vi "DblMonoPMDCurrentScanSM correction.vi"() -> ()   [LabVIEW 2009]
uses:
  <vilib>/DAQmx/create/channels.llb/DAQmx Create Channel (AI-Voltage-Basic).vi
  <vilib>/DAQmx/create/channels.llb/DAQmx Create Channel (AO-Voltage-Basic).vi
  <vilib>/DAQmx/write.llb/DAQmx Write (Analog DBL 1Chan 1Samp).vi
  <vilib>/DAQmx/read.llb/DAQmx Read (Analog 1D DBL 1Chan NSamp).vi
  <vilib>/DAQmx/configure/timing.llb/DAQmx Timing (Sample Clock).vi
  <vilib>/DAQmx/read.llb/DAQmx Read (Analog 1D DBL NChan 1Samp).vi
  <vilib>/DAQmx/write.llb/DAQmx Write (Analog 2D DBL NChan NSamp).vi
  <vilib>/Utility/file.llb/Write To Spreadsheet File (DBL).vi
  <vilib>/Analysis/NI_AALBase.lvlib
panel:
  out "element 2":dbl=0.0010963909721584337
  out "element":dbl=0.0027987340470992097
  out "number of samples written per channel":u32=999
  out "Waveform Chart  Y":dbl[](graph)=[0.0007739084085187373, 0.0007735634433916032, 0.0007732184782644691, 0.0007728735131373351, 0.0007725285480102011, 0.0007721835828830671, 0.0007718386177559331, 0.0007714936526287989, 0.0007711486875016649, 0.0007708037223745309, 0.0007704587572473969, 0.0007701137921202628, 0.0007697688269931288, 0.0007694238618659948, 0.0007690788967388608, 0.0007687339316117267, 0.0007683889664845927, 0.0007680440013574586, 0.0007676990362303246, 0.0007673540711031905, 0.0007670091059760565, 0.0007666641408489225, 0.0007663191757217885, 0.0007659742105946543, 0.0007656292454675203, 0.0007652842803403863, 0.0007649393152132523, 0.0007645943500861182, 0.0007642493849589842, 0.0007639044198318502, 0.0007635594547047162, 0.0007632144895775822, 0.000762869524450448, 0.000762524559323314, 0.00076217959419618, 0.000761834629069046, 0.0007614896639419119, 0.0007611446988147779, 0.0007607997336876438, 0.0007604547685605098, 0.0007601098034333757, 0.0007597648383062417, 0.0007594198731791077, 0.0007590749080519737, 0.0007587299429248396, 0.0007583849777977056, 0.0007580400126705716, 0.0007576950475434376, 0.0007573500824163034, 0.0007570051172891694, 0.0007566601521620354, 0.0007563151870349014, 0.0007559702219077673, 0.0007556252567806332, 0.0007552802916534992, 0.0007549353265263652, 0.0007545903613992311, 0.0007542453962720971, 0.0007539004311449631, 0.0007535554660178291, 0.0007532105008906951, 0.000752865535763561, 0.000752520570636427, 0.0007521756055092929, 0.0007518306403821589, 0.0007514856752550248, 0.0007511407101278908, 0.0007507957450007568, 0.0007504507798736228, 0.0007501058147464887, 0.0007497608496193547, 0.0007494158844922206, 0.0007490709193650866, 0.0007487259542379525, 0.0007483809891108185, 0.0007480360239836845, 0.0007476910588565505, 0.0007473460937294165, 0.0007470011286022824, 0.0007466561634751484, 0.0007463111983480143, 0.0007459662332208803, 0.0007456212680937462, 0.0007452763029666122, 0.0007449313378394782, 0.0007445863727123442, 0.00074424140758521, 0.000743896442458076, 0.000743551477330942, 0.000743206512203808, 0.0007428615470766739, 0.0007425165819495399, 0.0007421716168224059, 0.0007418266516952719, 0.0007414816865681378, 0.0007411367214410038, 0.0007407917563138697, 0.0007404467911867357, 0.0007401018260596016, 0.0007397568609324676, 0.0007394118958053336, 0.0007390669306781995, 0.0007387219655510654, 0.0007383770004239314, 0.0007380320352967974, 0.0007376870701696634, 0.0007373421050425294, 0.0007369971399153953, 0.0007366521747882613, 0.0007363072096611273, 0.0007359622445339933, 0.0007356172794068591, 0.0007352723142797251, 0.0007349273491525911, 0.0007345823840254571, 0.000734237418898323, 0.000733892453771189, 0.0007335474886440549, 0.0007332025235169209, 0.0007328575583897868, 0.0007325125932626528, 0.0007321676281355188, 0.0007318226630083848, 0.0007314776978812507, 0.0007311327327541167, 0.0007307877676269827, 0.0007304428024998486, 0.0007300978373727145, 0.0007297528722455805, 0.0007294079071184465, 0.0007290629419913125, 0.0007287179768641785, 0.0007283730117370443, 0.0007280280466099103, 0.0007276830814827763, 0.0007273381163556423, 0.0007269931512285082, 0.0007266481861013742, 0.0007263032209742402, 0.0007259582558471062, 0.0007256132907199721, 0.0007252683255928381, 0.000724923360465704, 0.00072457839533857, 0.0007242334302114359, 0.0007238884650843019, 0.0007235434999571679, 0.0007231985348300339, 0.0007228535697028998, 0.0007225086045757657, 0.0007221636394486317, 0.0007218186743214977, 0.0007214737091943636, 0.0007211287440672296, 0.0007207837789400956, 0.0007204388138129616, 0.0007200938486858276, 0.0007197488835586934, 0.0007194039184315594, 0.0007190589533044254, 0.0007187139881772914, 0.0007183690230501573, 0.0007180240579230233, 0.0007176790927958893, 0.0007173341276687553, 0.0007169891625416211, 0.0007166441974144871, 0.0007162992322873531, 0.0007159542671602191, 0.000715609302033085, 0.000715264336905951, 0.000714919371778817, 0.000714574406651683, 0.0007142294415245488, 0.0007138844763974148, 0.0007135395112702808, 0.0007131945461431468, 0.0007128495810160127, 0.0007125046158888787, 0.0007121596507617447, 0.0007118146856346106, 0.0007114697205074765, 0.0007111247553803425, 0.0007107797902532085, 0.0007104348251260745, 0.0007100898599989405, 0.0007097448948718064, 0.0007093999297446724, 0.0007090549646175384, 0.0007087099994904044, 0.0007083650343632702, 0.0007080200692361362, 0.0007076751041090022, 0.0007073301389818682, 0.0007069851738547341, 0.0007066402087276001, 0.000706295243600466, 0.000705950278473332, 0.0007056053133461979, 0.0007052603482190639, 0.0007049153830919299, 0.0007045704179647959, 0.0007042254528376618, 0.0007038804877105278, 0.0007035355225833938, 0.0007031905574562597, 0.0007028455923291256, 0.0007025006272019916, 0.0007021556620748576, 0.0007018106969477236, 0.0007014657318205896, 0.0007011207666934554, 0.0007007758015663214, 0.0007004308364391874, 0.0007000858713120534, 0.0006997409061849193, 0.0006993959410577853, 0.0006990509759306513, 0.0006987060108035173, 0.0006983610456763832, 0.0006980160805492492, 0.0006976711154221151, 0.0006973261502949811, 0.000696981185167847, 0.000696636220040713, 0.000696291254913579, 0.000695946289786445, 0.0006956013246593108, 0.0006952563595321769, 0.0006949113944050428, 0.0006945664292779088, 0.0006942214641507747, 0.0006938764990236407, 0.0006935315338965067, 0.0006931865687693727, 0.0006928416036422385, 0.0006924966385151046, 0.0006921516733879705, 0.0006918067082608365, 0.0006914617431337025, 0.0006911167780065684, 0.0006907718128794344, 0.0006904268477523004, 0.0006900818826251663, 0.0006897369174980323, 0.0006893919523708982, 0.0006890469872437642, 0.0006887020221166302, 0.0006883570569894961, 0.0006880120918623621, 0.0006876671267352281, 0.000687322161608094, 0.0006869771964809599, 0.0006866322313538259, 0.0006862872662266919, 0.0006859423010995579, 0.0006855973359724238, 0.0006852523708452898, 0.0006849074057181558, 0.0006845624405910217, 0.0006842174754638876, 0.0006838725103367536, 0.0006835275452096196, 0.0006831825800824856, 0.0006828376149553516, 0.0006824926498282175, 0.0006821476847010835, 0.0006818027195739495, 0.0006814577544468154, 0.0006811127893196814, 0.0006807678241925473, 0.0006804228590654133, 0.0006800778939382793, 0.0006797329288111451, 0.0006793879636840112, 0.0006790429985568771, 0.0006786980334297431, 0.000678353068302609, 0.000678008103175475, 0.000677663138048341, 0.000677318172921207, 0.000676973207794073, 0.0006766282426669389, 0.0006762832775398049, 0.0006759383124126708, 0.0006755933472855367, 0.0006752483821584027, 0.0006749034170312687, 0.0006745584519041347, 0.0006742134867770005, 0.0006738685216498666, 0.0006735235565227325, 0.0006731785913955985, 0.0006728336262684645, 0.0006724886611413304, 0.0006721436960141964, 0.0006717987308870624, 0.0006714537657599284, 0.0006711088006327942, 0.0006707638355056603, 0.0006704188703785262, 0.0006700739052513922, 0.0006697289401242581, 0.0006693839749971241, 0.0006690390098699901, 0.0006686940447428561, 0.0006683490796157219, 0.000668004114488588, 0.0006676591493614539, 0.0006673141842343199, 0.0006669692191071858, 0.0006666242539800518, 0.0006662792888529178, 0.0006659343237257838, 0.0006655893585986496, 0.0006652443934715157, 0.0006648994283443816, 0.0006645544632172476, 0.0006642094980901136, 0.0006638645329629795, 0.0006635195678358455, 0.0006631746027087115, 0.0006628296375815774, 0.0006624846724544433, 0.0006621397073273093, 0.0006617947422001753, 0.0006614497770730413, 0.0006611048119459072, 0.0006607598468187732, 0.0006604148816916392, 0.0006600699165645051, 0.000659724951437371, 0.000659379986310237, 0.000659035021183103, 0.000658690056055969, 0.000658345090928835, 0.0006580001258017009, 0.0006576551606745669, 0.0006573101955474328, 0.0006569652304202987, 0.0006566202652931647, 0.0006562753001660307, 0.0006559303350388967, 0.0006555853699117627, 0.0006552404047846286, 0.0006548954396574946, 0.0006545504745303605, 0.0006542055094032265, 0.0006538605442760924, 0.0006535155791489584, 0.0006531706140218244, 0.0006528256488946904, 0.0006524806837675562, 0.0006521357186404223, 0.0006517907535132882, 0.0006514457883861542, 0.0006511008232590201, 0.0006507558581318861, 0.0006504108930047521, 0.0006500659278776181, 0.000649720962750484, 0.00064937599762335, 0.000649031032496216, 0.0006486860673690819, 0.0006483411022419479, 0.0006479961371148138, 0.0006476511719876798, 0.0006473062068605458, 0.0006469612417334117, 0.0006466162766062777, 0.0006462713114791436, 0.0006459263463520096, 0.0006455813812248756, 0.0006452364160977415, 0.0006448914509706075, 0.0006445464858434735, 0.0006442015207163395, 0.0006438565555892053, 0.0006435115904620714, 0.0006431666253349373, 0.0006428216602078033, 0.0006424766950806692, 0.0006421317299535352, 0.0006417867648264012, 0.0006414417996992672, 0.000641096834572133, 0.0006407518694449991, 0.000640406904317865, 0.000640061939190731, 0.000639716974063597, 0.0006393720089364629, 0.0006390270438093289, 0.0006386820786821949, 0.0006383371135550608, 0.0006379921484279268, 0.0006376471833007927, 0.0006373022181736587, 0.0006369572530465247, 0.0006366122879193906, 0.0006362673227922566, 0.0006359223576651226, 0.0006355773925379885, 0.0006352324274108544, 0.0006348874622837204, 0.0006345424971565864, 0.0006341975320294524, 0.0006338525669023183, 0.0006335076017751843, 0.0006331626366480503, 0.0006328176715209162, 0.0006324727063937821, 0.0006321277412666481, 0.0006317827761395141, 0.0006314378110123801, 0.000631092845885246, 0.000630747880758112, 0.000630402915630978, 0.0006300579505038439, 0.0006297129853767099, 0.0006293680202495758, 0.0006290230551224418, 0.0006286780899953078, 0.0006283331248681738, 0.0006279881597410396, 0.0006276431946139057, 0.0006272982294867716, 0.0006269532643596376, 0.0006266082992325035, 0.0006262633341053695, 0.0006259183689782355, 0.0006255734038511015, 0.0006252284387239673, 0.0006248834735968334, 0.0006245385084696993, 0.0006241935433425653, 0.0006238485782154312, 0.0006235036130882972, 0.0006231586479611632, 0.0006228136828340292, 0.000622468717706895, 0.0006221237525797611, 0.000621778787452627, 0.000621433822325493, 0.000621088857198359, 0.0006207438920712249, 0.0006203989269440909, 0.0006200539618169569, 0.0006197089966898228, 0.0006193640315626887, 0.0006190190664355547, 0.0006186741013084207, 0.0006183291361812867, 0.0006179841710541526, 0.0006176392059270186, 0.0006172942407998846, 0.0006169492756727506, 0.0006166043105456164, 0.0006162593454184825, 0.0006159143802913484, 0.0006155694151642144, 0.0006152244500370803, 0.0006148794849099463, 0.0006145345197828123, 0.0006141895546556783, 0.0006138445895285441, 0.0006134996244014102, 0.0006131546592742761, 0.0006128096941471421, 0.000612464729020008, 0.000612119763892874, 0.00061177479876574, 0.000611429833638606, 0.0006110848685114719, 0.0006107399033843378, 0.0006103949382572038, 0.0006100499731300698, 0.0006097050080029358, 0.0006093600428758017, 0.0006090150777486677, 0.0006086701126215337, 0.0006083251474943996, 0.0006079801823672655, 0.0006076352172401315, 0.0006072902521129975, 0.0006069452869858635, 0.0006066003218587294, 0.0006062553567315954, 0.0006059103916044614, 0.0006055654264773273, 0.0006052204613501932, 0.0006048754962230592, 0.0006045305310959252, 0.0006041855659687912, 0.0006038406008416572, 0.000603495635714523, 0.0006031506705873891, 0.000602805705460255, 0.000602460740333121, 0.0006021157752059869, 0.0006017708100788529, 0.0006014258449517189, 0.0006010808798245849, 0.0006007359146974508, 0.0006003909495703168, 0.0006000459844431828, 0.0005997010193160487, 0.0005993560541889146, 0.0005990110890617806, 0.0005986661239346466, 0.0005983211588075126, 0.0005979761936803785, 0.0005976312285532445, 0.0005972862634261105, 0.0005969412982989764, 0.0005965963331718423, 0.0005962513680447083, 0.0005959064029175743, 0.0005955614377904403, 0.0005952164726633063, 0.0005948715075361721, 0.0005945265424090382, 0.0005941815772819041, 0.0005938366121547701, 0.000593491647027636, 0.000593146681900502, 0.000592801716773368, 0.000592456751646234, 0.0005921117865190998, 0.0005917668213919659, 0.0005914218562648318, 0.0005910768911376978, 0.0005907319260105637, 0.0005903869608834297, 0.0005900419957562957, 0.0005896970306291617, 0.0005893520655020275, 0.0005890071003748936, 0.0005886621352477595, 0.0005883171701206255, 0.0005879722049934914, 0.0005876272398663574, 0.0005872822747392234, 0.0005869373096120894, 0.0005865923444849552, 0.0005862473793578212, 0.0005859024142306872, 0.0005855574491035532, 0.0005852124839764192, 0.0005848675188492851, 0.0005845225537221511, 0.0005841775885950171, 0.000583832623467883, 0.0005834876583407489, 0.0005831426932136149, 0.0005827977280864809, 0.0005824527629593469, 0.0005821077978322128, 0.0005817628327050788, 0.0005814178675779448, 0.0005810729024508107, 0.0005807279373236766, 0.0005803829721965426, 0.0005800380070694086, 0.0005796930419422746, 0.0005793480768151405, 0.0005790031116880065, 0.0005786581465608725, 0.0005783131814337384, 0.0005779682163066043, 0.0005776232511794703, 0.0005772782860523363, 0.0005769333209252023, 0.0005765883557980683, 0.0005762433906709341, 0.0005758984255438002, 0.0005755534604166661, 0.0005752084952895321, 0.000574863530162398, 0.000574518565035264, 0.00057417359990813, 0.000573828634780996, 0.0005734836696538618, 0.0005731387045267279, 0.0005727937393995939, 0.0005724487742724598, 0.0005721038091453257, 0.0005717588440181917, 0.0005714138788910577, 0.0005710689137639237, 0.0005707239486367895, 0.0005703789835096556, 0.0005700340183825215, 0.0005696890532553875, 0.0005693440881282534, 0.0005689991230011194, 0.0005686541578739854, 0.0005683091927468514, 0.0005679642276197174, 0.0005676192624925832, 0.0005672742973654493, 0.0005669293322383152, 0.0005665843671111812, 0.0005662394019840471, 0.0005658944368569131, 0.0005655494717297791, 0.0005652045066026451, 0.0005648595414755109, 0.000564514576348377, 0.0005641696112212429, 0.0005638246460941089, 0.0005634796809669748, 0.0005631347158398408, 0.0005627897507127068, 0.0005624447855855728, 0.0005620998204584386, 0.0005617548553313047, 0.0005614098902041706, 0.0005610649250770366, 0.0005607199599499026, 0.0005603749948227685, 0.0005600300296956345, 0.0005596850645685005, 0.0005593400994413664, 0.0005589951343142323, 0.0005586501691870983, 0.0005583052040599643, 0.0005579602389328303, 0.0005576152738056962, 0.0005572703086785622, 0.0005569253435514282, 0.0005565803784242941, 0.00055623541329716, 0.000555890448170026, 0.000555545483042892, 0.000555200517915758, 0.0005548555527886239, 0.0005545105876614899, 0.0005541656225343559, 0.0005538206574072218, 0.0005534756922800877, 0.0005531307271529537, 0.0005527857620258197, 0.0005524407968986857, 0.0005520958317715517, 0.0005517508666444175, 0.0005514059015172836, 0.0005510609363901495, 0.0005507159712630155, 0.0005503710061358814, 0.0005500260410087474, 0.0005496810758816134, 0.0005493361107544794, 0.0005489911456273452, 0.0005486461805002113, 0.0005483012153730772, 0.0005479562502459432, 0.0005476112851188091, 0.0005472663199916751, 0.0005469213548645411, 0.0005465763897374071, 0.0005462314246102729, 0.000545886459483139, 0.0005455414943560049, 0.0005451965292288709, 0.0005448515641017368, 0.0005445065989746028, 0.0005441616338474688, 0.0005438166687203348, 0.0005434717035932006, 0.0005431267384660666, 0.0005427817733389326, 0.0005424368082117986, 0.0005420918430846646, 0.0005417468779575305, 0.0005414019128303965, 0.0005410569477032625, 0.0005407119825761285, 0.0005403670174489943, 0.0005400220523218604, 0.0005396770871947263, 0.0005393321220675923, 0.0005389871569404582, 0.0005386421918133242, 0.0005382972266861902, 0.0005379522615590561, 0.000537607296431922, 0.000537262331304788, 0.000536917366177654, 0.00053657240105052, 0.0005362274359233859, 0.0005358824707962519, 0.0005355375056691179, 0.0005351925405419839, 0.0005348475754148497, 0.0005345026102877157, 0.0005341576451605817, 0.0005338126800334477, 0.0005334677149063137, 0.0005331227497791796, 0.0005327777846520456, 0.0005324328195249116, 0.0005320878543977775, 0.0005317428892706434, 0.0005313979241435094, 0.0005310529590163754, 0.0005307079938892414, 0.0005303630287621073, 0.0005300180636349733, 0.0005296730985078393, 0.0005293281333807052, 0.0005289831682535711, 0.0005286382031264371, 0.0005282932379993031, 0.0005279482728721691, 0.000527603307745035, 0.000527258342617901, 0.000526913377490767, 0.0005265684123636329, 0.0005262234472364988, 0.0005258784821093648, 0.0005255335169822308, 0.0005251885518550968, 0.0005248435867279628, 0.0005244986216008286, 0.0005241536564736947, 0.0005238086913465606, 0.0005234637262194266, 0.0005231187610922925, 0.0005227737959651585, 0.0005224288308380245, 0.0005220838657108905, 0.0005217389005837563, 0.0005213939354566224, 0.0005210489703294883, 0.0005207040052023543, 0.0005203590400752202, 0.0005200140749480862, 0.0005196691098209522, 0.0005193241446938182, 0.000518979179566684, 0.0005186342144395501, 0.0005182892493124161, 0.000517944284185282, 0.000517599319058148, 0.0005172543539310139, 0.0005169093888038799, 0.0005165644236767459, 0.0005162194585496117, 0.0005158744934224777, 0.0005155295282953437, 0.0005151845631682097, 0.0005148395980410757, 0.0005144946329139416, 0.0005141496677868076, 0.0005138047026596736, 0.0005134597375325396, 0.0005131147724054054, 0.0005127698072782715, 0.0005124248421511374, 0.0005120798770240034, 0.0005117349118968693, 0.0005113899467697353, 0.0005110449816426013, 0.0005107000165154672, 0.0005103550513883331, 0.0005100100862611991, 0.0005096651211340651, 0.0005093201560069311, 0.000508975190879797, 0.000508630225752663, 0.000508285260625529, 0.000507940295498395, 0.0005075953303712608, 0.0005072503652441268, 0.0005069054001169928, 0.0005065604349898588, 0.0005062154698627248, 0.0005058705047355906, 0.0005055255396084567, 0.0005051805744813226, 0.0005048356093541886, 0.0005044906442270545, 0.0005041456790999205, 0.0005038007139727865, 0.0005034557488456525, 0.0005031107837185184, 0.0005027658185913844, 0.0005024208534642504, 0.0005020758883371163, 0.0005017309232099822, 0.0005013859580828482, 0.0005010409929557142, 0.0005006960278285802, 0.0005003510627014461, 0.000500006097574312, 0.0004996611324471781, 0.000499316167320044, 0.00049897120219291, 0.0004986262370657759, 0.0004982812719386419, 0.0004979363068115079, 0.0004975913416843739, 0.0004972463765572397, 0.0004969014114301058, 0.0004965564463029717, 0.0004962114811758377, 0.0004958665160487036, 0.0004955215509215696, 0.0004951765857944356, 0.0004948316206673016, 0.0004944866555401674, 0.0004941416904130335, 0.0004937967252858994, 0.0004934517601587654, 0.0004931067950316313, 0.0004927618299044973, 0.0004924168647773633, 0.0004920718996502293, 0.0004917269345230951, 0.0004913819693959611, 0.0004910370042688271, 0.0004906920391416931, 0.000490347074014559, 0.000490002108887425, 0.000489657143760291, 0.000489312178633157, 0.0004889672135060228, 0.0004886222483788888, 0.00048827728325175486, 0.0004879323181246208, 0.00048758735299748676, 0.00048724238787035273, 0.0004868974227432187, 0.0004865524576160847, 0.0004862074924889506, 0.00048586252736181653, 0.00048551756223468256, 0.0004851725971075485, 0.00048482763198041446, 0.00048448266685328044, 0.00048413770172614636, 0.0004837927365990124, 0.0004834477714718783, 0.00048310280634474424, 0.0004827578412176102, 0.0004824128760904762, 0.00048206791096334217, 0.00048172294583620815, 0.00048137798070907407, 0.0004810330155819401, 0.000480688050454806, 0.00048034308532767195, 0.0004799981202005379, 0.0004796531550734039, 0.0004793081899462699, 0.00047896322481913586, 0.0004786182596920018, 0.0004782732945648678, 0.00047792832943773373, 0.00047758336431059966, 0.00047723839918346563, 0.0004768934340563316, 0.0004765484689291976, 0.00047620350380206357, 0.0004758585386749295, 0.0004755135735477954, 0.00047516860842066144, 0.00047482364329352736, 0.00047447867816639334, 0.0004741337130392593, 0.0004737887479121253, 0.0004734437827849913, 0.0004730988176578572, 0.0004727538525307231, 0.00047240888740358915, 0.00047206392227645507, 0.00047171895714932105, 0.000471373992022187, 0.000471029026895053, 0.000470684061767919, 0.0004703390966407849, 0.0004699941315136508, 0.00046964916638651686, 0.0004693042012593828, 0.00046895923613224876, 0.00046861427100511473, 0.0004682693058779807, 0.0004679243407508467, 0.0004675793756237126, 0.00046723441049657853, 0.0004668894453694445, 0.00046654448024231054, 0.00046619951511517647, 0.00046585454998804244, 0.0004655095848609084, 0.0004651646197337744, 0.0004648196546066404, 0.0004644746894795063, 0.0004641297243523722, 0.00046378475922523825, 0.0004634397940981042, 0.00046309482897097015, 0.00046274986384383613, 0.0004624048987167021, 0.0004620599335895681, 0.000461714968462434, 0.00046137000333529993, 0.00046102503820816596, 0.0004606800730810319, 0.00046033510795389786, 0.00045999014282676384, 0.0004596451776996298, 0.0004593002125724958, 0.0004589552474453617, 0.00045861028231822764, 0.0004582653171910936, 0.0004579203520639596, 0.00045757538693682557, 0.00045723042180969154, 0.00045688545668255747, 0.0004565404915554235, 0.0004561955264282894, 0.00045585056130115534, 0.0004555055961740214, 0.0004551606310468873, 0.0004548156659197533, 0.00045447070079261925, 0.0004541257356654852, 0.0004537807705383511, 0.0004534358054112171, 0.00045309084028408316, 0.0004527458751569491, 0.000452400910029815, 0.000452055944902681, 0.00045171097977554696, 0.0004513660146484129, 0.0004510210495212788, 0.0004506760843941448, 0.00045033111926701076, 0.0004499861541398768, 0.0004496411890127427, 0.0004492962238856087, 0.00044895125875847467, 0.0004486062936313406, 0.0004482613285042065, 0.0004479163633770725, 0.00044757139824993847, 0.0004472264331228045, 0.0004468814679956704, 0.0004465365028685364, 0.0004461915377414024, 0.0004458465726142683, 0.0004455016074871342, 0.0004451566423600002, 0.0004448116772328662, 0.0004444667121057322, 0.00044412174697859813, 0.0004437767818514641, 0.0004434318167243301, 0.000443086851597196, 0.00044274188647006193, 0.0004423969213429279, 0.0004420519562157939, 0.0004417069910886598, 0.00044136202596152584, 0.0004410170608343918, 0.0004406720957072578, 0.0004403271305801237, 0.00043998216545298964, 0.0004396372003258556, 0.0004392922351987216, 0.0004389472700715875, 0.00043860230494445355, 0.0004382573398173195, 0.0004379123746901855, 0.0004375674095630514, 0.00043722244443591734, 0.0004368774793087833, 0.0004365325141816493, 0.0004361875490545153, 0.0004358425839273813, 0.00043549761880024723, 0.0004351526536731132, 0.0004348076885459792, 0.0004344627234188451, 0.00043411775829171103, 0.000433772793164577, 0.000433427828037443, 0.0004330828629103089, 0.00043273789778317494, 0.0004323929326560409, 0.0004320479675289069, 0.0004317030024017728, 0.00043135803727463874, 0.0004310130721475047, 0.0004306681070203707, 0.0004303231418932366, 0.00042997817676610265, 0.0004296332116389686, 0.0004292882465118346]
  out "initial y":dbl=0.0007739084085187373
  out "Final Y":dbl=0.0004292882465118346
  out "Waveform Chart X":dbl[](graph)=[0.003443699175398357, 0.0034438293846314775, 0.003443959593864598, 0.0034440898030977185, 0.0034442200123308386, 0.003444350221563959, 0.0034444804307970796, 0.0034446106400301997, 0.00344474084926332, 0.0034448710584964407, 0.0034450012677295612, 0.0034451314769626813, 0.003445261686195802, 0.0034453918954289223, 0.0034455221046620424, 0.003445652313895163, 0.0034457825231282834, 0.0034459127323614035, 0.003446042941594524, 0.0034461731508276445, 0.003446303360060765, 0.003446433569293885, 0.0034465637785270056, 0.003446693987760126, 0.003446824196993246, 0.0034469544062263667, 0.003447084615459487, 0.0034472148246926073, 0.0034473450339257278, 0.0034474752431588483, 0.003447605452391969, 0.003447735661625089, 0.0034478658708582094, 0.00344799608009133, 0.00344812628932445, 0.0034482564985575705, 0.003448386707790691, 0.0034485169170238115, 0.0034486471262569316, 0.003448777335490052, 0.0034489075447231726, 0.0034490377539562926, 0.003449167963189413, 0.0034492981724225337, 0.0034494283816556537, 0.0034495585908887742, 0.0034496888001218948, 0.0034498190093550153, 0.0034499492185881353, 0.003450079427821256, 0.0034502096370543764, 0.0034503398462874964, 0.003450470055520617, 0.0034506002647537374, 0.0034507304739868575, 0.003450860683219978, 0.0034509908924530985, 0.003451121101686219, 0.003451251310919339, 0.0034513815201524596, 0.00345151172938558, 0.0034516419386187, 0.0034517721478518207, 0.0034519023570849412, 0.0034520325663180613, 0.003452162775551182, 0.0034522929847843023, 0.003452423194017423, 0.003452553403250543, 0.0034526836124836634, 0.003452813821716784, 0.003452944030949904, 0.0034530742401830245, 0.003453204449416145, 0.0034533346586492655, 0.0034534648678823856, 0.003453595077115506, 0.0034537252863486266, 0.0034538554955817467, 0.003453985704814867, 0.0034541159140479877, 0.0034542461232811078, 0.0034543763325142283, 0.003454506541747349, 0.0034546367509804693, 0.0034547669602135894, 0.00345489716944671, 0.0034550273786798304, 0.0034551575879129505, 0.003455287797146071, 0.0034554180063791915, 0.0034555482156123116, 0.003455678424845432, 0.0034558086340785526, 0.003455938843311673, 0.003456069052544793, 0.0034561992617779137, 0.003456329471011034, 0.0034564596802441542, 0.0034565898894772747, 0.0034567200987103953, 0.0034568503079435158, 0.003456980517176636, 0.0034571107264097563, 0.003457240935642877, 0.003457371144875997, 0.0034575013541091174, 0.003457631563342238, 0.003457761772575358, 0.0034578919818084785, 0.003458022191041599, 0.0034581524002747195, 0.0034582826095078396, 0.00345841281874096, 0.0034585430279740806, 0.0034586732372072007, 0.0034588034464403212, 0.0034589336556734417, 0.003459063864906562, 0.0034591940741396823, 0.003459324283372803, 0.0034594544926059233, 0.0034595847018390434, 0.003459714911072164, 0.0034598451203052844, 0.0034599753295384045, 0.003460105538771525, 0.0034602357480046455, 0.0034603659572377656, 0.003460496166470886, 0.0034606263757040066, 0.003460756584937127, 0.003460886794170247, 0.0034610170034033677, 0.003461147212636488, 0.0034612774218696083, 0.0034614076311027288, 0.0034615378403358493, 0.00346166804956897, 0.00346179825880209, 0.0034619284680352104, 0.003462058677268331, 0.003462188886501451, 0.0034623190957345715, 0.003462449304967692, 0.003462579514200812, 0.0034627097234339326, 0.003462839932667053, 0.0034629701419001736, 0.0034631003511332937, 0.003463230560366414, 0.0034633607695995347, 0.0034634909788326547, 0.0034636211880657753, 0.0034637513972988958, 0.003463881606532016, 0.0034640118157651363, 0.003464142024998257, 0.0034642722342313774, 0.0034644024434644974, 0.003464532652697618, 0.0034646628619307385, 0.0034647930711638585, 0.003464923280396979, 0.0034650534896300995, 0.00346518369886322, 0.00346531390809634, 0.0034654441173294606, 0.003465574326562581, 0.003465704535795701, 0.0034658347450288217, 0.0034659649542619422, 0.0034660951634950623, 0.003466225372728183, 0.0034663555819613033, 0.003466485791194424, 0.003466616000427544, 0.0034667462096606644, 0.003466876418893785, 0.003467006628126905, 0.0034671368373600255, 0.003467267046593146, 0.003467397255826266, 0.0034675274650593866, 0.003467657674292507, 0.0034677878835256276, 0.0034679180927587477, 0.003468048301991868, 0.0034681785112249887, 0.0034683087204581088, 0.0034684389296912293, 0.00346856913892435, 0.00346869934815747, 0.0034688295573905904, 0.003468959766623711, 0.0034690899758568314, 0.0034692201850899515, 0.003469350394323072, 0.0034694806035561925, 0.0034696108127893126, 0.003469741022022433, 0.0034698712312555536, 0.003470001440488674, 0.003470131649721794, 0.0034702618589549147, 0.003470392068188035, 0.0034705222774211552, 0.0034706524866542758, 0.0034707826958873963, 0.0034709129051205163, 0.003471043114353637, 0.0034711733235867574, 0.003471303532819878, 0.003471433742052998, 0.0034715639512861184, 0.003471694160519239, 0.003471824369752359, 0.0034719545789854795, 0.0034720847882186, 0.00347221499745172, 0.0034723452066848406, 0.003472475415917961, 0.0034726056251510816, 0.0034727358343842017, 0.0034728660436173222, 0.0034729962528504427, 0.003473126462083563, 0.0034732566713166833, 0.003473386880549804, 0.003473517089782924, 0.0034736472990160444, 0.003473777508249165, 0.0034739077174822854, 0.0034740379267154055, 0.003474168135948526, 0.0034742983451816465, 0.0034744285544147666, 0.003474558763647887, 0.0034746889728810076, 0.003474819182114128, 0.003474949391347248, 0.0034750796005803687, 0.003475209809813489, 0.0034753400190466093, 0.00347547022827973, 0.0034756004375128503, 0.0034757306467459704, 0.003475860855979091, 0.0034759910652122114, 0.003476121274445332, 0.003476251483678452, 0.0034763816929115725, 0.003476511902144693, 0.003476642111377813, 0.0034767723206109336, 0.003476902529844054, 0.003477032739077174, 0.0034771629483102947, 0.003477293157543415, 0.0034774233667765357, 0.0034775535760096558, 0.0034776837852427763, 0.0034778139944758968, 0.003477944203709017, 0.0034780744129421374, 0.003478204622175258, 0.0034783348314083784, 0.0034784650406414984, 0.003478595249874619, 0.0034787254591077395, 0.0034788556683408595, 0.00347898587757398, 0.0034791160868071005, 0.0034792462960402206, 0.003479376505273341, 0.0034795067145064616, 0.003479636923739582, 0.0034797671329727022, 0.0034798973422058227, 0.0034800275514389432, 0.0034801577606720633, 0.003480287969905184, 0.0034804181791383043, 0.0034805483883714244, 0.003480678597604545, 0.0034808088068376654, 0.003480939016070786, 0.003481069225303906, 0.0034811994345370265, 0.003481329643770147, 0.003481459853003267, 0.0034815900622363876, 0.003481720271469508, 0.0034818504807026286, 0.0034819806899357487, 0.003482110899168869, 0.0034822411084019897, 0.00348237131763511, 0.0034825015268682303, 0.003482631736101351, 0.003482761945334471, 0.0034828921545675914, 0.003483022363800712, 0.0034831525730338324, 0.0034832827822669525, 0.003483412991500073, 0.0034835432007331935, 0.0034836734099663136, 0.003483803619199434, 0.0034839338284325546, 0.0034840640376656747, 0.003484194246898795, 0.0034843244561319157, 0.003484454665365036, 0.0034845848745981563, 0.0034847150838312768, 0.0034848452930643973, 0.0034849755022975173, 0.003485105711530638, 0.0034852359207637584, 0.0034853661299968784, 0.003485496339229999, 0.0034856265484631195, 0.00348575675769624, 0.00348588696692936, 0.0034860171761624805, 0.003486147385395601, 0.003486277594628721, 0.0034864078038618416, 0.003486538013094962, 0.0034866682223280827, 0.0034867984315612027, 0.0034869286407943232, 0.0034870588500274437, 0.003487189059260564, 0.0034873192684936843, 0.003487449477726805, 0.003487579686959925, 0.0034877098961930454, 0.003487840105426166, 0.0034879703146592864, 0.0034881005238924065, 0.003488230733125527, 0.0034883609423586475, 0.0034884911515917676, 0.003488621360824888, 0.0034887515700580086, 0.0034888817792911287, 0.003489011988524249, 0.0034891421977573697, 0.00348927240699049, 0.0034894026162236103, 0.003489532825456731, 0.0034896630346898513, 0.0034897932439229714, 0.003489923453156092, 0.0034900536623892124, 0.0034901838716223325, 0.003490314080855453, 0.0034904442900885735, 0.003490574499321694, 0.003490704708554814, 0.0034908349177879346, 0.003490965127021055, 0.003491095336254175, 0.0034912255454872957, 0.003491355754720416, 0.0034914859639535367, 0.0034916161731866568, 0.0034917463824197773, 0.0034918765916528978, 0.003492006800886018, 0.0034921370101191384, 0.003492267219352259, 0.003492397428585379, 0.0034925276378184994, 0.00349265784705162, 0.0034927880562847405, 0.0034929182655178605, 0.003493048474750981, 0.0034931786839841016, 0.0034933088932172216, 0.003493439102450342, 0.0034935693116834626, 0.0034936995209165827, 0.0034938297301497032, 0.0034939599393828237, 0.0034940901486159442, 0.0034942203578490643, 0.003494350567082185, 0.0034944807763153053, 0.0034946109855484254, 0.003494741194781546, 0.0034948714040146664, 0.0034950016132477865, 0.003495131822480907, 0.0034952620317140275, 0.003495392240947148, 0.003495522450180268, 0.0034956526594133886, 0.003495782868646509, 0.003495913077879629, 0.0034960432871127497, 0.00349617349634587, 0.0034963037055789907, 0.003496433914812111, 0.0034965641240452313, 0.003496694333278352, 0.003496824542511472, 0.0034969547517445924, 0.003497084960977713, 0.003497215170210833, 0.0034973453794439535, 0.003497475588677074, 0.0034976057979101945, 0.0034977360071433146, 0.003497866216376435, 0.0034979964256095556, 0.0034981266348426757, 0.003498256844075796, 0.0034983870533089167, 0.0034985172625420368, 0.0034986474717751573, 0.0034987776810082778, 0.0034989078902413983, 0.0034990380994745184, 0.003499168308707639, 0.0034992985179407594, 0.0034994287271738794, 0.003499558936407, 0.0034996891456401205, 0.003499819354873241, 0.003499949564106361, 0.0035000797733394816, 0.003500209982572602, 0.003500340191805722, 0.0035004704010388426, 0.003500600610271963, 0.0035007308195050832, 0.0035008610287382037, 0.0035009912379713242, 0.0035011214472044448, 0.003501251656437565, 0.0035013818656706853, 0.003501512074903806, 0.003501642284136926, 0.0035017724933700464, 0.003501902702603167, 0.003502032911836287, 0.0035021631210694075, 0.003502293330302528, 0.0035024235395356485, 0.0035025537487687686, 0.003502683958001889, 0.0035028141672350096, 0.0035029443764681297, 0.00350307458570125, 0.0035032047949343707, 0.003503335004167491, 0.0035034652134006113, 0.003503595422633732, 0.0035037256318668523, 0.0035038558410999724, 0.003503986050333093, 0.0035041162595662134, 0.0035042464687993335, 0.003504376678032454, 0.0035045068872655745, 0.003504637096498695, 0.003504767305731815, 0.0035048975149649356, 0.003505027724198056, 0.003505157933431176, 0.0035052881426642967, 0.003505418351897417, 0.0035055485611305373, 0.0035056787703636578, 0.0035058089795967783, 0.0035059391888298988, 0.003506069398063019, 0.0035061996072961394, 0.00350632981652926, 0.00350646002576238, 0.0035065902349955005, 0.003506720444228621, 0.003506850653461741, 0.0035069808626948615, 0.003507111071927982, 0.0035072412811611026, 0.0035073714903942226, 0.003507501699627343, 0.0035076319088604637, 0.0035077621180935837, 0.0035078923273267042, 0.0035080225365598247, 0.003508152745792945, 0.0035082829550260653, 0.003508413164259186, 0.0035085433734923063, 0.0035086735827254264, 0.003508803791958547, 0.0035089340011916674, 0.0035090642104247875, 0.003509194419657908, 0.0035093246288910285, 0.003509454838124149, 0.003509585047357269, 0.0035097152565903896, 0.00350984546582351, 0.00350997567505663, 0.0035101058842897507, 0.003510236093522871, 0.0035103663027559913, 0.003510496511989112, 0.0035106267212222323, 0.003510756930455353, 0.003510887139688473, 0.0035110173489215934, 0.003511147558154714, 0.003511277767387834, 0.0035114079766209545, 0.003511538185854075, 0.003511668395087195, 0.0035117986043203156, 0.003511928813553436, 0.0035120590227865566, 0.0035121892320196767, 0.003512319441252797, 0.0035124496504859177, 0.0035125798597190378, 0.0035127100689521583, 0.0035128402781852788, 0.003512970487418399, 0.0035131006966515194, 0.00351323090588464, 0.0035133611151177604, 0.0035134913243508805, 0.003513621533584001, 0.0035137517428171215, 0.0035138819520502415, 0.003514012161283362, 0.0035141423705164826, 0.003514272579749603, 0.003514402788982723, 0.0035145329982158437, 0.003514663207448964, 0.0035147934166820842, 0.0035149236259152047, 0.0035150538351483252, 0.0035151840443814453, 0.003515314253614566, 0.0035154444628476863, 0.003515574672080807, 0.003515704881313927, 0.0035158350905470474, 0.003515965299780168, 0.003516095509013288, 0.0035162257182464085, 0.003516355927479529, 0.003516486136712649, 0.0035166163459457696, 0.00351674655517889, 0.0035168767644120106, 0.0035170069736451307, 0.003517137182878251, 0.0035172673921113717, 0.003517397601344492, 0.0035175278105776123, 0.003517658019810733, 0.0035177882290438533, 0.0035179184382769734, 0.003518048647510094, 0.0035181788567432144, 0.0035183090659763345, 0.003518439275209455, 0.0035185694844425755, 0.0035186996936756956, 0.003518829902908816, 0.0035189601121419366, 0.003519090321375057, 0.003519220530608177, 0.0035193507398412977, 0.003519480949074418, 0.0035196111583075383, 0.0035197413675406588, 0.0035198715767737793, 0.0035200017860068994, 0.00352013199524002, 0.0035202622044731404, 0.003520392413706261, 0.003520522622939381, 0.0035206528321725015, 0.003520783041405622, 0.003520913250638742, 0.0035210434598718626, 0.003521173669104983, 0.003521303878338103, 0.0035214340875712236, 0.003521564296804344, 0.0035216945060374647, 0.0035218247152705847, 0.0035219549245037052, 0.0035220851337368258, 0.003522215342969946, 0.0035223455522030663, 0.003522475761436187, 0.0035226059706693074, 0.0035227361799024274, 0.003522866389135548, 0.0035229965983686684, 0.0035231268076017885, 0.003523257016834909, 0.0035233872260680295, 0.0035235174353011496, 0.00352364764453427, 0.0035237778537673906, 0.003523908063000511, 0.003524038272233631, 0.0035241684814667517, 0.0035242986906998722, 0.0035244288999329923, 0.003524559109166113, 0.0035246893183992333, 0.0035248195276323534, 0.003524949736865474, 0.0035250799460985944, 0.003525210155331715, 0.003525340364564835, 0.0035254705737979555, 0.003525600783031076, 0.003525730992264196, 0.0035258612014973166, 0.003525991410730437, 0.003526121619963557, 0.0035262518291966777, 0.003526382038429798, 0.0035265122476629187, 0.0035266424568960388, 0.0035267726661291593, 0.00352690287536228, 0.0035270330845954, 0.0035271632938285204, 0.003527293503061641, 0.0035274237122947614, 0.0035275539215278815, 0.003527684130761002, 0.0035278143399941225, 0.0035279445492272426, 0.003528074758460363, 0.0035282049676934836, 0.0035283351769266036, 0.003528465386159724, 0.0035285955953928447, 0.003528725804625965, 0.0035288560138590852, 0.0035289862230922057, 0.0035291164323253263, 0.0035292466415584463, 0.003529376850791567, 0.0035295070600246873, 0.0035296372692578074, 0.003529767478490928, 0.0035298976877240484, 0.003530027896957169, 0.003530158106190289, 0.0035302883154234095, 0.00353041852465653, 0.00353054873388965, 0.0035306789431227706, 0.003530809152355891, 0.0035309393615890116, 0.0035310695708221317, 0.0035311997800552522, 0.0035313299892883727, 0.003531460198521493, 0.0035315904077546133, 0.003531720616987734, 0.003531850826220854, 0.0035319810354539744, 0.003532111244687095, 0.0035322414539202154, 0.0035323716631533355, 0.003532501872386456, 0.0035326320816195765, 0.0035327622908526966, 0.003532892500085817, 0.0035330227093189376, 0.0035331529185520577, 0.003533283127785178, 0.0035334133370182987, 0.003533543546251419, 0.0035336737554845393, 0.0035338039647176598, 0.0035339341739507803, 0.0035340643831839004, 0.003534194592417021, 0.0035343248016501414, 0.003534455010883262, 0.003534585220116382, 0.0035347154293495025, 0.003534845638582623, 0.003534975847815743, 0.0035351060570488636, 0.003535236266281984, 0.003535366475515104, 0.0035354966847482247, 0.003535626893981345, 0.0035357571032144657, 0.0035358873124475857, 0.0035360175216807063, 0.0035361477309138268, 0.003536277940146947, 0.0035364081493800673, 0.003536538358613188, 0.003536668567846308, 0.0035367987770794284, 0.003536928986312549, 0.0035370591955456695, 0.0035371894047787895, 0.00353731961401191, 0.0035374498232450305, 0.0035375800324781506, 0.003537710241711271, 0.0035378404509443916, 0.0035379706601775117, 0.003538100869410632, 0.0035382310786437527, 0.0035383612878768732, 0.0035384914971099933, 0.003538621706343114, 0.0035387519155762343, 0.0035388821248093544, 0.003539012334042475, 0.0035391425432755954, 0.003539272752508716, 0.003539402961741836, 0.0035395331709749565, 0.003539663380208077, 0.003539793589441197, 0.0035399237986743176, 0.003540054007907438, 0.003540184217140558, 0.0035403144263736787, 0.003540444635606799, 0.0035405748448399197, 0.0035407050540730398, 0.0035408352633061603, 0.003540965472539281, 0.003541095681772401, 0.0035412258910055214, 0.003541356100238642, 0.003541486309471762, 0.0035416165187048825, 0.003541746727938003, 0.0035418769371711235, 0.0035420071464042436, 0.003542137355637364, 0.0035422675648704846, 0.0035423977741036046, 0.003542527983336725, 0.0035426581925698457, 0.0035427884018029657, 0.0035429186110360862, 0.0035430488202692068, 0.0035431790295023273, 0.0035433092387354473, 0.003543439447968568, 0.0035435696572016884, 0.0035436998664348084, 0.003543830075667929, 0.0035439602849010494, 0.00354409049413417, 0.00354422070336729, 0.0035443509126004105, 0.003544481121833531, 0.003544611331066651, 0.0035447415402997716, 0.003544871749532892, 0.003545001958766012, 0.0035451321679991327, 0.0035452623772322532, 0.0035453925864653737, 0.003545522795698494, 0.0035456530049316143, 0.003545783214164735, 0.003545913423397855, 0.0035460436326309754, 0.003546173841864096, 0.003546304051097216, 0.0035464342603303365, 0.003546564469563457, 0.0035466946787965775, 0.0035468248880296976, 0.003546955097262818, 0.0035470853064959386, 0.0035472155157290587, 0.003547345724962179, 0.0035474759341952997, 0.00354760614342842, 0.0035477363526615403, 0.003547866561894661, 0.0035479967711277813, 0.0035481269803609014, 0.003548257189594022, 0.0035483873988271424, 0.0035485176080602625, 0.003548647817293383, 0.0035487780265265035, 0.003548908235759624, 0.003549038444992744, 0.0035491686542258646, 0.003549298863458985, 0.003549429072692105, 0.0035495592819252257, 0.003549689491158346, 0.0035498197003914662, 0.0035499499096245868, 0.0035500801188577073, 0.0035502103280908278, 0.003550340537323948, 0.0035504707465570684, 0.003550600955790189, 0.003550731165023309, 0.0035508613742564294, 0.00355099158348955, 0.00355112179272267, 0.0035512520019557905, 0.003551382211188911, 0.0035515124204220315, 0.0035516426296551516, 0.003551772838888272, 0.0035519030481213926, 0.0035520332573545127, 0.0035521634665876332, 0.0035522936758207537, 0.0035524238850538742, 0.0035525540942869943, 0.003552684303520115, 0.0035528145127532353, 0.0035529447219863554, 0.003553074931219476, 0.0035532051404525964, 0.0035533353496857165, 0.003553465558918837, 0.0035535957681519575, 0.003553725977385078, 0.003553856186618198, 0.0035539863958513186, 0.003554116605084439, 0.003554246814317559, 0.0035543770235506797, 0.0035545072327838, 0.0035546374420169203, 0.003554767651250041, 0.0035548978604831613, 0.003555028069716282, 0.003555158278949402, 0.0035552884881825224, 0.003555418697415643, 0.003555548906648763, 0.0035556791158818835, 0.003555809325115004, 0.003555939534348124, 0.0035560697435812446, 0.003556199952814365, 0.0035563301620474856, 0.0035564603712806057, 0.003556590580513726, 0.0035567207897468467, 0.0035568509989799667, 0.0035569812082130873, 0.0035571114174462078, 0.0035572416266793283, 0.0035573718359124483, 0.003557502045145569, 0.0035576322543786894, 0.0035577624636118094, 0.00355789267284493, 0.0035580228820780505, 0.0035581530913111705, 0.003558283300544291, 0.0035584135097774115, 0.003558543719010532, 0.003558673928243652, 0.0035588041374767726, 0.003558934346709893, 0.0035590645559430132, 0.0035591947651761337, 0.0035593249744092542, 0.0035594551836423743, 0.003559585392875495, 0.0035597156021086153, 0.003559845811341736, 0.003559976020574856, 0.0035601062298079764, 0.003560236439041097, 0.003560366648274217, 0.0035604968575073375, 0.003560627066740458, 0.003560757275973578, 0.0035608874852066986, 0.003561017694439819, 0.0035611479036729396, 0.0035612781129060597, 0.00356140832213918, 0.0035615385313723007, 0.0035616687406054208, 0.0035617989498385413, 0.003561929159071662, 0.0035620593683047823, 0.0035621895775379024, 0.003562319786771023, 0.0035624499960041434, 0.0035625802052372635, 0.003562710414470384, 0.0035628406237035045, 0.0035629708329366246, 0.003563101042169745, 0.0035632312514028656, 0.003563361460635986, 0.003563491669869106, 0.0035636218791022267, 0.003563752088335347, 0.0035638822975684673, 0.0035640125068015878, 0.0035641427160347083, 0.0035642729252678288, 0.003564403134500949, 0.0035645333437340694, 0.00356466355296719, 0.00356479376220031, 0.0035649239714334304, 0.003565054180666551, 0.003565184389899671, 0.0035653145991327915, 0.003565444808365912, 0.0035655750175990326, 0.0035657052268321526, 0.003565835436065273, 0.0035659656452983936, 0.0035660958545315137, 0.0035662260637646342, 0.0035663562729977547, 0.003566486482230875, 0.0035666166914639953, 0.003566746900697116, 0.0035668771099302363, 0.0035670073191633564, 0.003567137528396477, 0.0035672677376295974, 0.0035673979468627175, 0.003567528156095838, 0.0035676583653289585, 0.003567788574562079, 0.003567918783795199, 0.0035680489930283196, 0.00356817920226144, 0.00356830941149456, 0.0035684396207276807, 0.003568569829960801, 0.0035687000391939213, 0.003568830248427042, 0.0035689604576601623, 0.003569090666893283, 0.003569220876126403, 0.0035693510853595234, 0.003569481294592644, 0.003569611503825764, 0.0035697417130588845, 0.003569871922292005, 0.003570002131525125, 0.0035701323407582456, 0.003570262549991366, 0.0035703927592244866, 0.0035705229684576067, 0.003570653177690727, 0.0035707833869238477, 0.0035709135961569678, 0.0035710438053900883, 0.0035711740146232088, 0.003571304223856329, 0.0035714344330894494, 0.00357156464232257, 0.0035716948515556904, 0.0035718250607888104, 0.003571955270021931, 0.0035720854792550515, 0.0035722156884881715, 0.003572345897721292, 0.0035724761069544126, 0.0035726063161875326, 0.003572736525420653, 0.0035728667346537736, 0.003572996943886894, 0.0035731271531200142, 0.0035732573623531347, 0.0035733875715862552, 0.0035735177808193753, 0.003573647990052496, 0.0035737781992856163]
  out "initial x":dbl=0.003443699175398357
  out "Final x":dbl=0.0035737781992856163
  in  "Volts/pixel":dbl=-0.0002
  out "Xin":dbl=0.0034436991753983574
  out "Yin":dbl=0.0007739084085187373
  in  "Correction":dbl[][](array[numeric])=[[460.0, 480.0, 1.0, -5.0], [480.0, 490.0, 4.0, -6.0], [490.0, 510.0, 4.0, -6.0], [510.0, 530.0, 7.0, -4.0], [530.0, 550.0, 6.0, -4.0], [550.0, 570.0, 11.0, -2.0], [570.0, 590.0, 18.0, 1.0], [590.0, 610.0, 16.0, 1.0], [610.0, 630.0, 22.0, 4.0], [630.0, 650.0, 25.0, 4.0], [650.0, 670.0, 31.0, 4.0], [670.0, 690.0, 24.0, 6.0], [690.0, 710.0, 25.0, 5.0], [710.0, 730.0, 23.0, 3.0], [730.0, 750.0, 19.0, 1.0], [750.0, 780.0, 9.0, 1.0], [780.0, 800.0, 12.0, 0.0]]
  in  "Scan mirrors out":tag="Dev1/ao1:0"
  in  "Scan Mirrors in":tag="Dev1/ai1:2"
  in  "Voltage B":dbl min=-10.0 max=10.0 step=0.1 format="%0.2f"
  in  "Voltage A":dbl min=-10.0 max=10.0 step=0.1 format="%0.2f"
  in  "Output B":tag="Dev1/ao3"
  in  "Output A":tag="Dev1/ao2"
  in  "Input Channel":tag="Dev1/ai6"
  in  "Current":bool
  in  "Power":bool=TRUE
  out "ScanGraph":cluster{dbl[], dbl[]}(graph)={[459.986, 464.987, 469.988, 474.99, 479.99, 484.99, 489.99, 494.99, 499.989, 504.988, 509.986, 514.984, 519.999, 524.996, 529.993, 534.99, 539.986, 544.998, 549.994, 554.99, 559.984, 564.995, 569.99, 574.983, 579.993, 584.986, 589.994, 594.986, 599.995, 604.986, 609.993, 614.983, 619.99, 624.995, 629.985, 634.99, 639.994, 644.999, 649.986, 654.989, 659.992, 664.994, 669.996, 674.997, 679.998, 684.998, 689.983, 694.998, 699.997, 704.996, 709.994, 714.991, 719.988, 724.985, 729.997, 734.993, 739.988, 744.999], [2.1099248219999993e-07, 4.841876133e-06, -1.5273329160000004e-06, 1.7982357982999998e-06, 1.6874433263e-06, 1.7260287571e-06, 4.2421699291e-06, 1.0175213299e-05, 6.336555329000002e-07, 2.8867754744e-06, 9.7345900059e-06, 2.0786917676e-06, 1.262283729e-06, 7.0713391289999995e-06, 2.155351334e-06, -1.245506316000002e-07, 2.1544726345e-06, 2.2136387822e-06, -3.900836119999998e-07, -1.0242116113e-06, 4.19034681275e-06, 1.1503179743e-06, 6.3705236194e-06, 2.431987241e-06, 3.2818190054e-06, 2.2443169879999996e-06, -1.7280163039999998e-07, 3.4131044219999993e-07, -3.1544439536e-06, 4.743758288999999e-07, 2.61580934e-06, 5.132718029e-06, 2.411577974e-06, 2.1582370003e-06, 1.4940037116e-06, -8.682694599999961e-09, 1.1422522415e-06, 1.0737787442000001e-06, -2.239742121e-07, 1.0586110429e-06, 1.0709150784e-06, 1.2884574339000001e-06, 1.0348154043e-06, 4.847385682e-07, 5.49520904e-07, 1.7452527669999997e-07, 4.2117633290000003e-07, 1.07371440189e-06, 2.3799586880999999e-07, 5.871614649e-07, 9.4995538737e-07, -2.8246480500000006e-08, 7.429808617e-08, 6.2026416241e-07, 3.0612814373e-07, 7.033739084e-07, 9.849100580000001e-08, 5.508379621499999e-07]}
  in  "Sensitivity":dbl=1e-09 caption="(A/V)" format="%#_6p"
  out "Readout":dbl=4.29846551e-07 format="%^#_9e"
  in  "Scan Save Path":path
  in  "On":bool=TRUE
  out "Waveform Chart":dbl(graph)=4.29846551e-07
  in  "Save":bool
  in  "Exit":bool
  in  "STOP":bool
  in  "Step Time (sec)":dbl=1.0 min=0.001 max=300.0 step=0.001 format="%.3f"
  in  "Step Size (nm)":dbl=5.0 min=0.1 max=100.0 step=0.1 format="%.1f"
  in  "End":dbl=800.0 min=0.0 max=2000.0 step=0.1 format="%.1f"
  in  "Start":dbl=460.0 min=0.0 max=2000.0 step=0.1 format="%.1f"
  in  "Scan":bool
  in  "Up":bool=TRUE caption="Down"
  in  "Increment (nm)":dbl=10.0 min=0.1 max=2000.0 step=0.1 format="%.1f"
  in  "PMD Settings":T1={"Beam Diameter (mm)"=4.0, "BWIn"=0, "Averaging Rate"=300, "Auto Range"=TRUE} {"Averaging Rate" min=33 max=5000 step=1; "BWIn" items=["HIGH", "LOW"]; "Beam Diameter (mm)" min=1.0 max=9.0 step=0.5}
  in  "Step":bool
  out "Busy":bool
  in  "Send Command":bool
  in  "Command":u16(ring)=1 items=["nm", "goto", "nm/min", "VIS grating", "IR grating"]
  in  "Wavelength (nm)":dbl=745.0 min=0.0 max=2000.0 step=0.1 format="%.1f"
  in  "Scan Speed (nm/min)":dbl=100.0 min=1.0 max=500.0 step=0.1 format="%.1f"
  out "Done?":string="  ok\r\n"
  in  "Send Question":bool
  in  "Ask?":u16(ring) items=["?nm", "?nm/min", "?grating", "?turret", "?gratings"]
  in  "Zero?":bool
  out "PM Error log":string
  out "AUTO?":bool
  out "Zero Value":dbl format="%#.3p"
  out "Rng":string
  in  "Range":i16=1 min=1 max=6 step=1
  in  "Mono Port":refnum<visa-resource-name>="COM11"
  out "IDN String":string="Thorlabs,PM100USB,P2000362,1.3.0\n"
  out "Sensor SN":string="10061433"
  out "Sensor Name":string="S120C"
  out "Reply":string=" 744.999 nm  ok\r\n" caption="Mono Response"
  # "Range Settings"
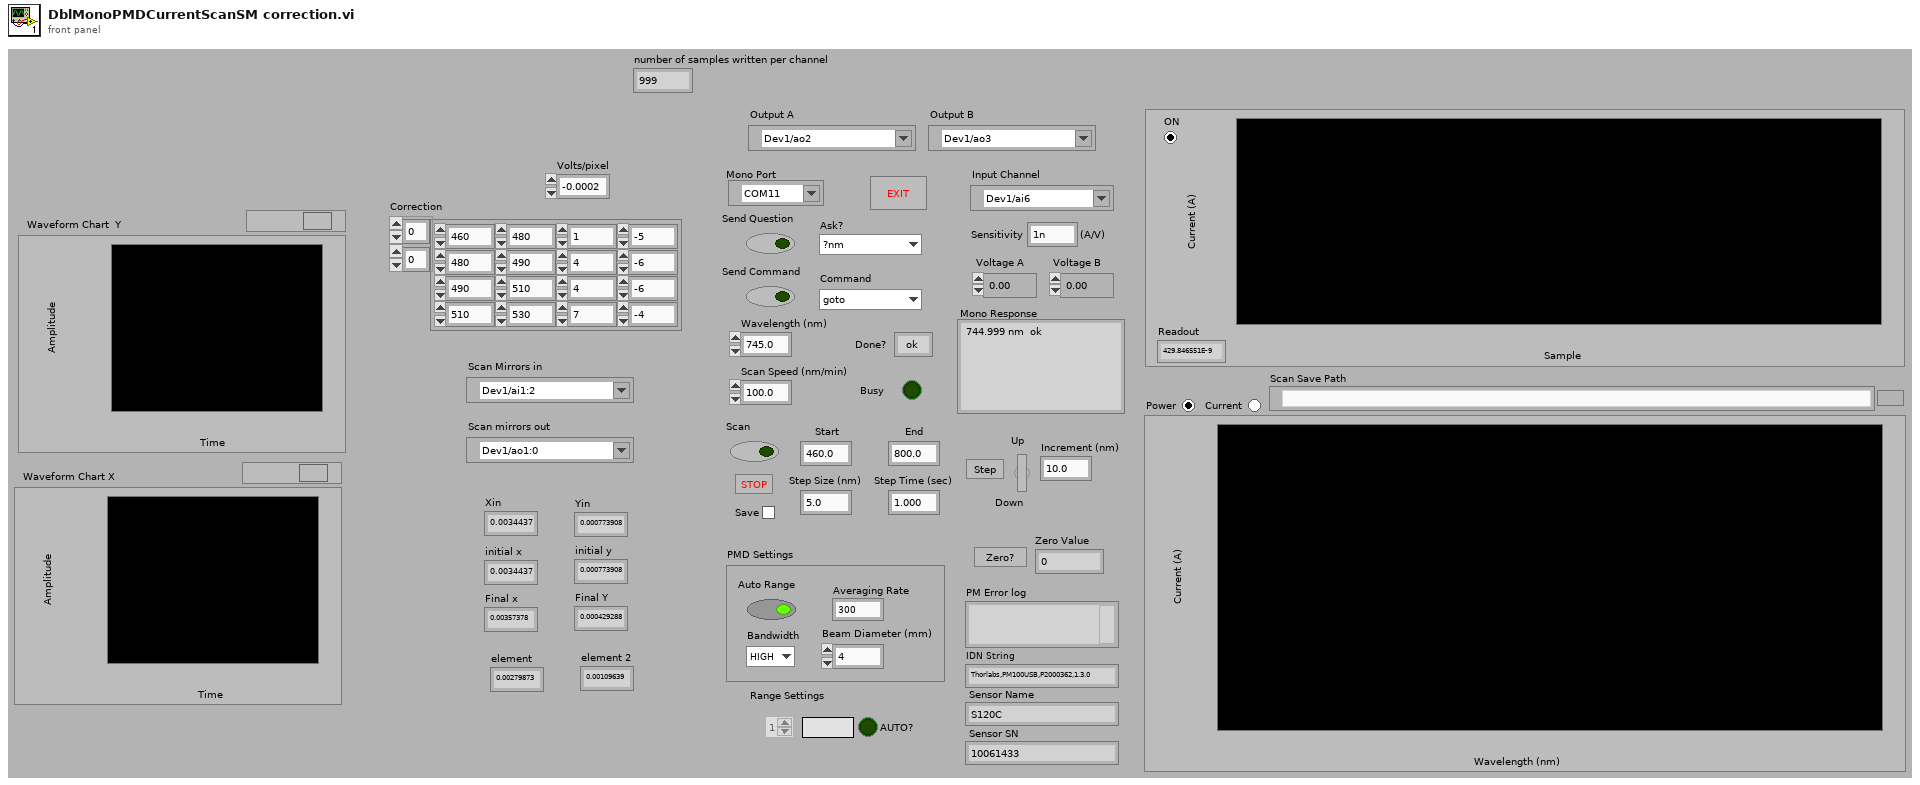
[diagram p1: front panel]
types:
  T1 = cluster{"Beam Diameter (mm)":dbl, "BWIn":u16, "Averaging Rate":i32, "Auto Range":bool}
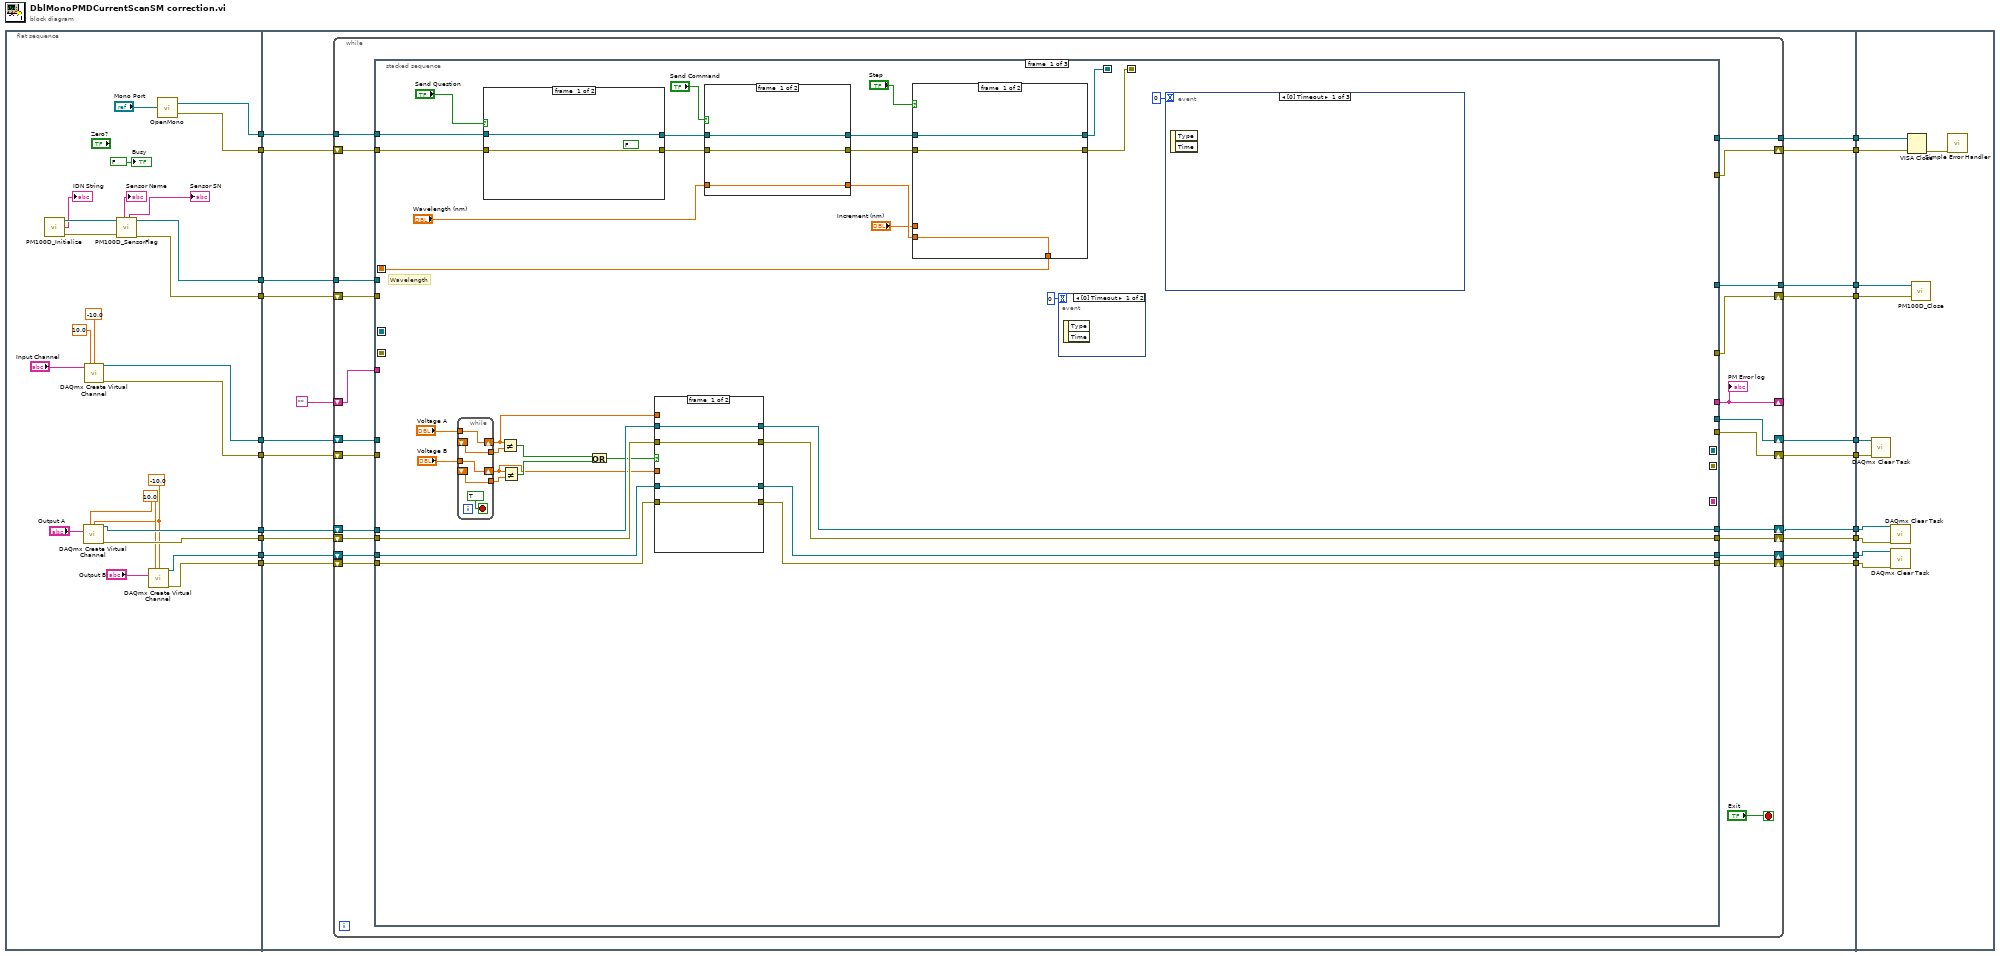
[diagram p0: block diagram]
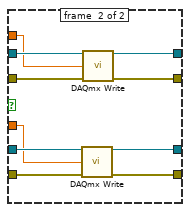
[diagram p2: hidden frame]
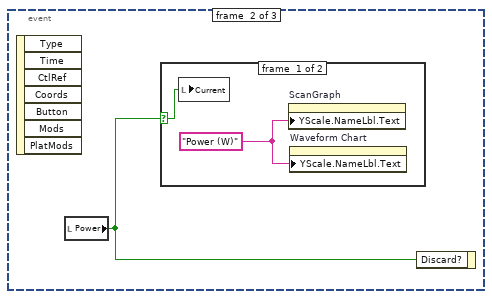
[diagram p3: hidden frame]
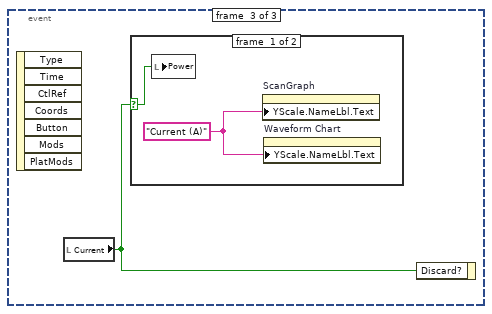
[diagram p5: hidden frame]
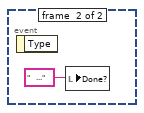
[diagram p7: hidden frame]
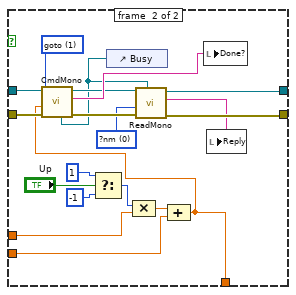
[diagram p8: hidden frame]
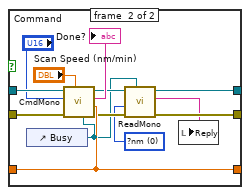
[diagram p9: hidden frame]
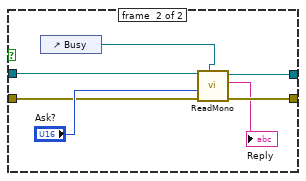
[diagram p10: hidden frame]
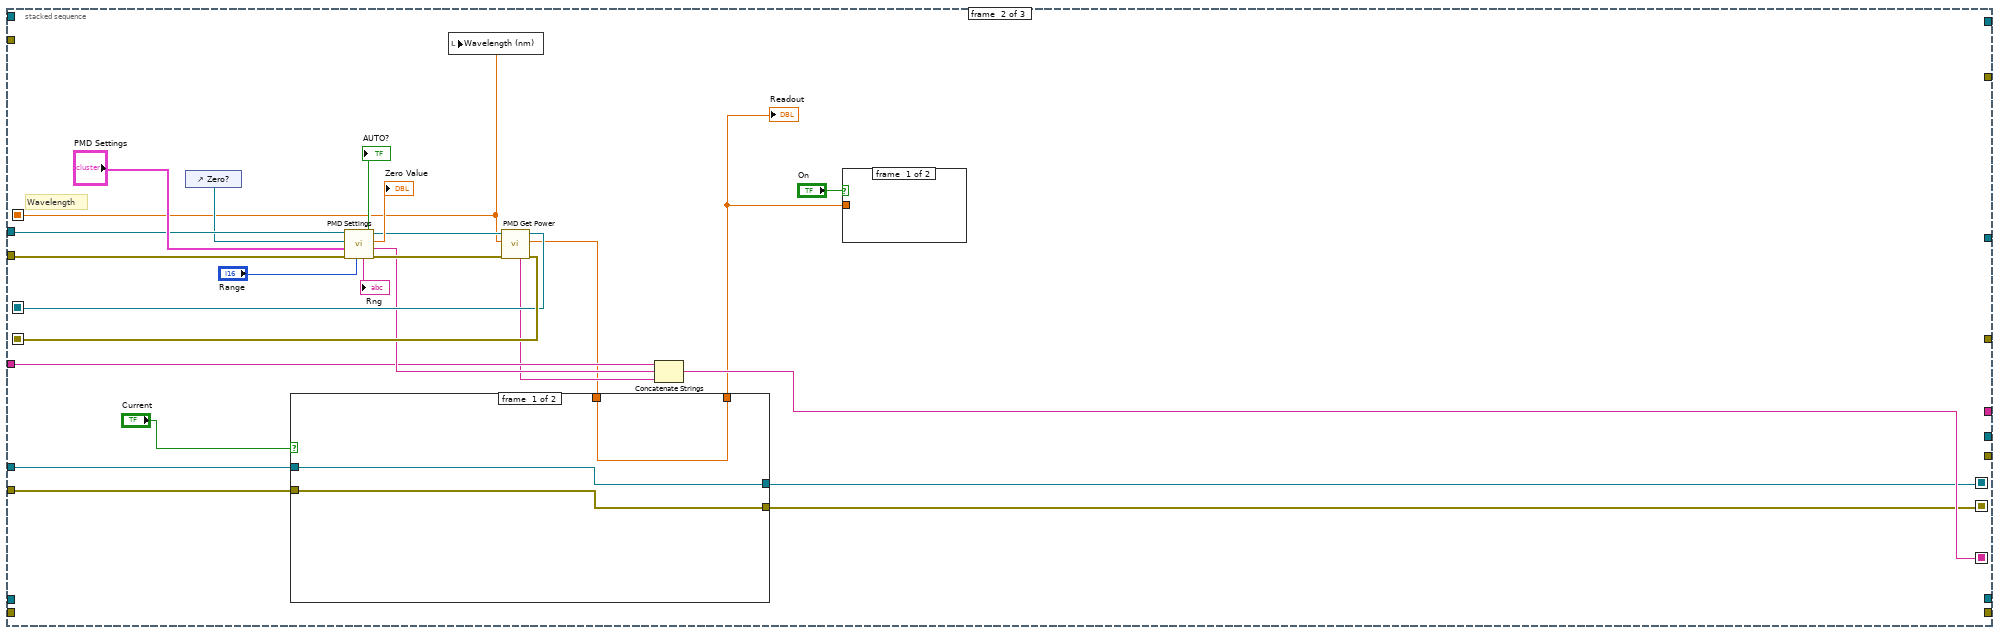
[diagram p11: hidden frame]
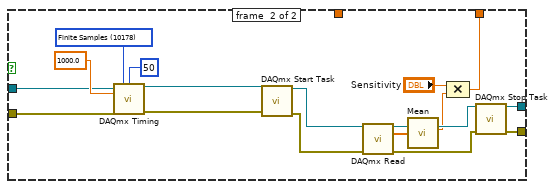
[diagram p12: hidden frame]
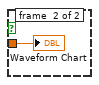
[diagram p13: hidden frame]
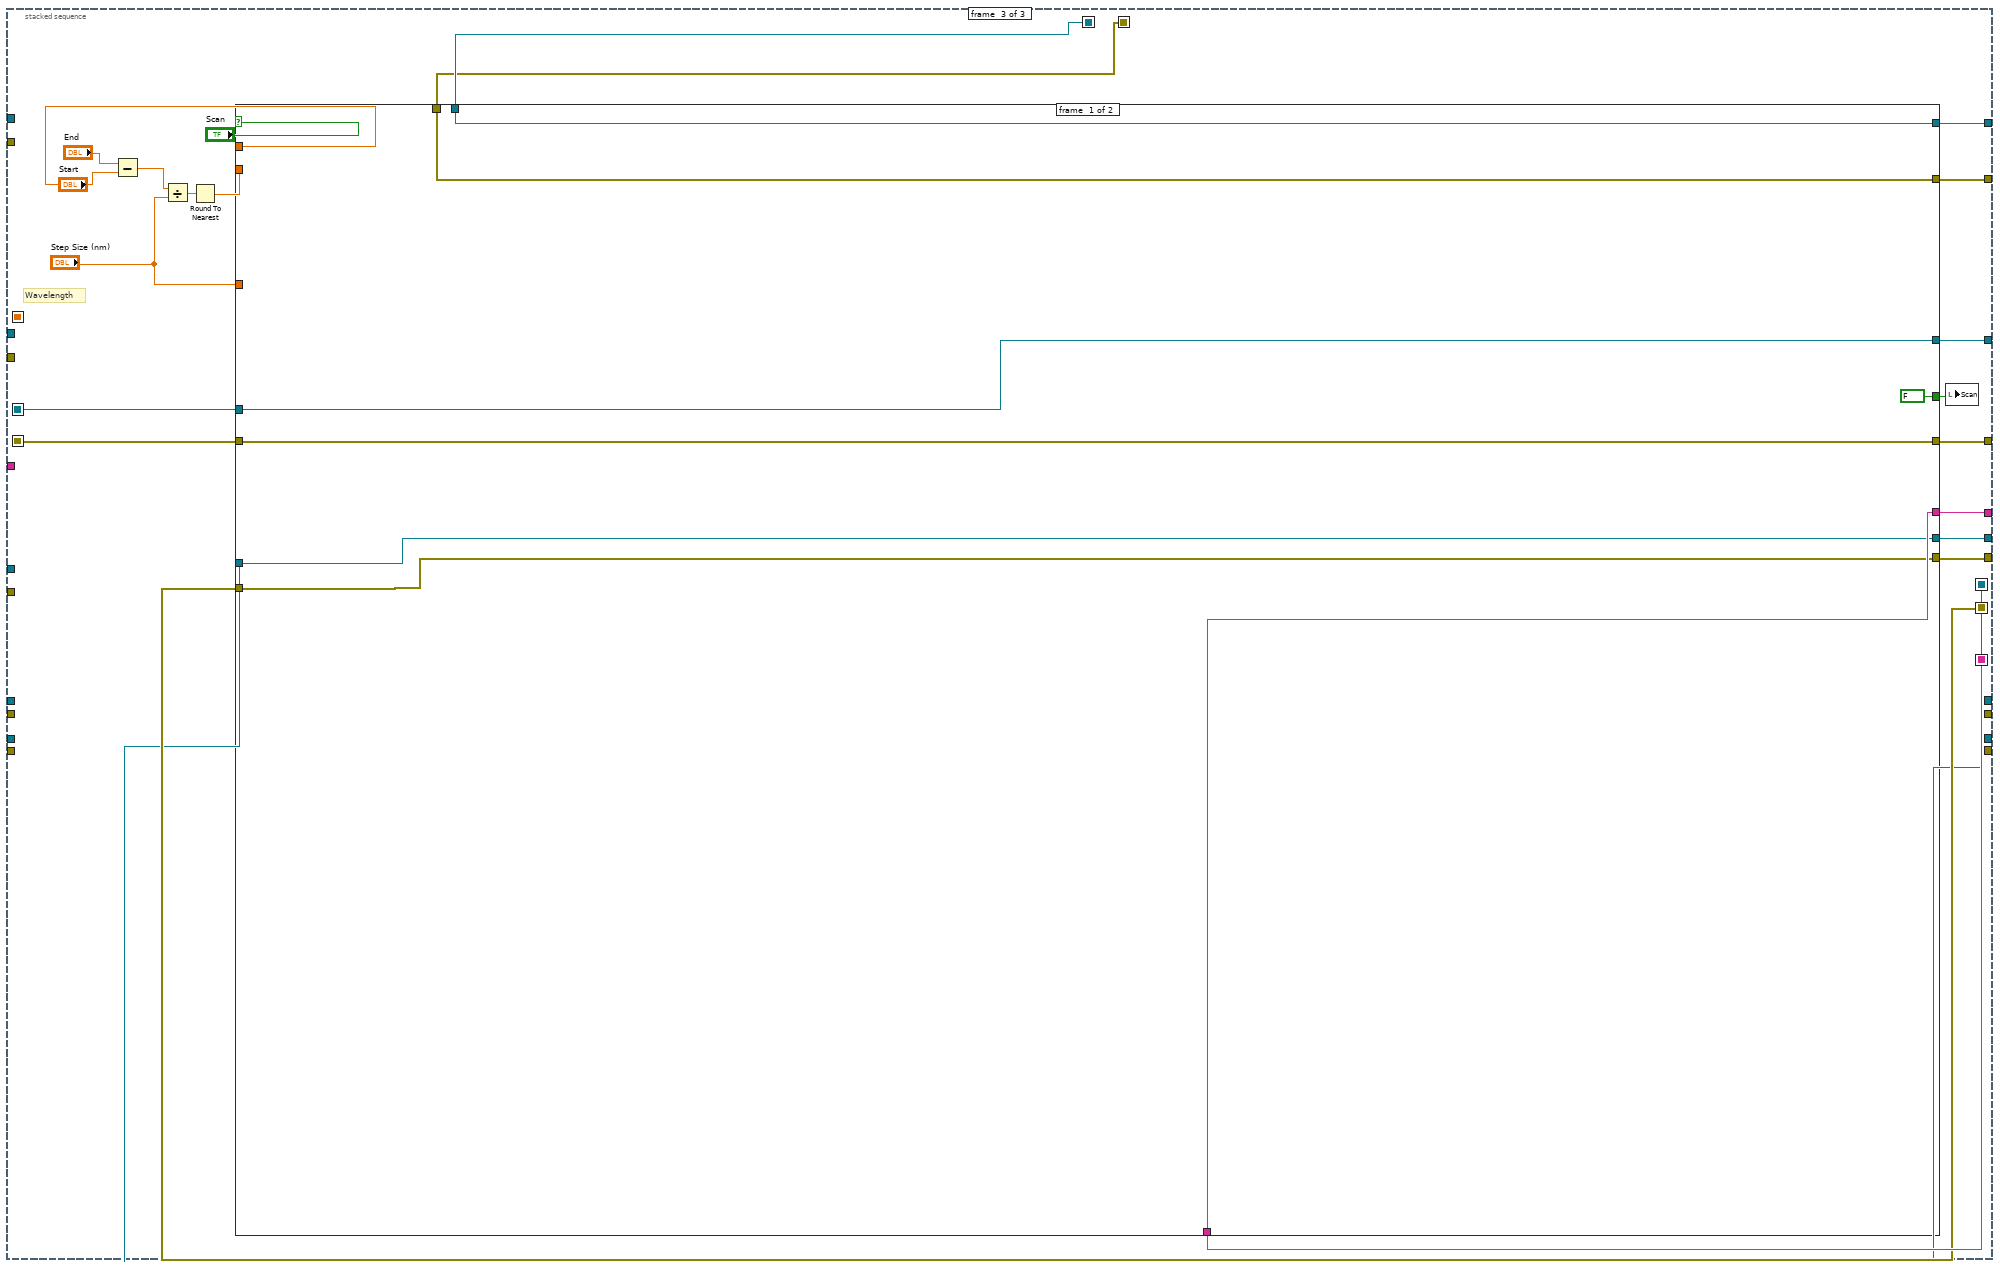
[diagram p14: hidden frame]
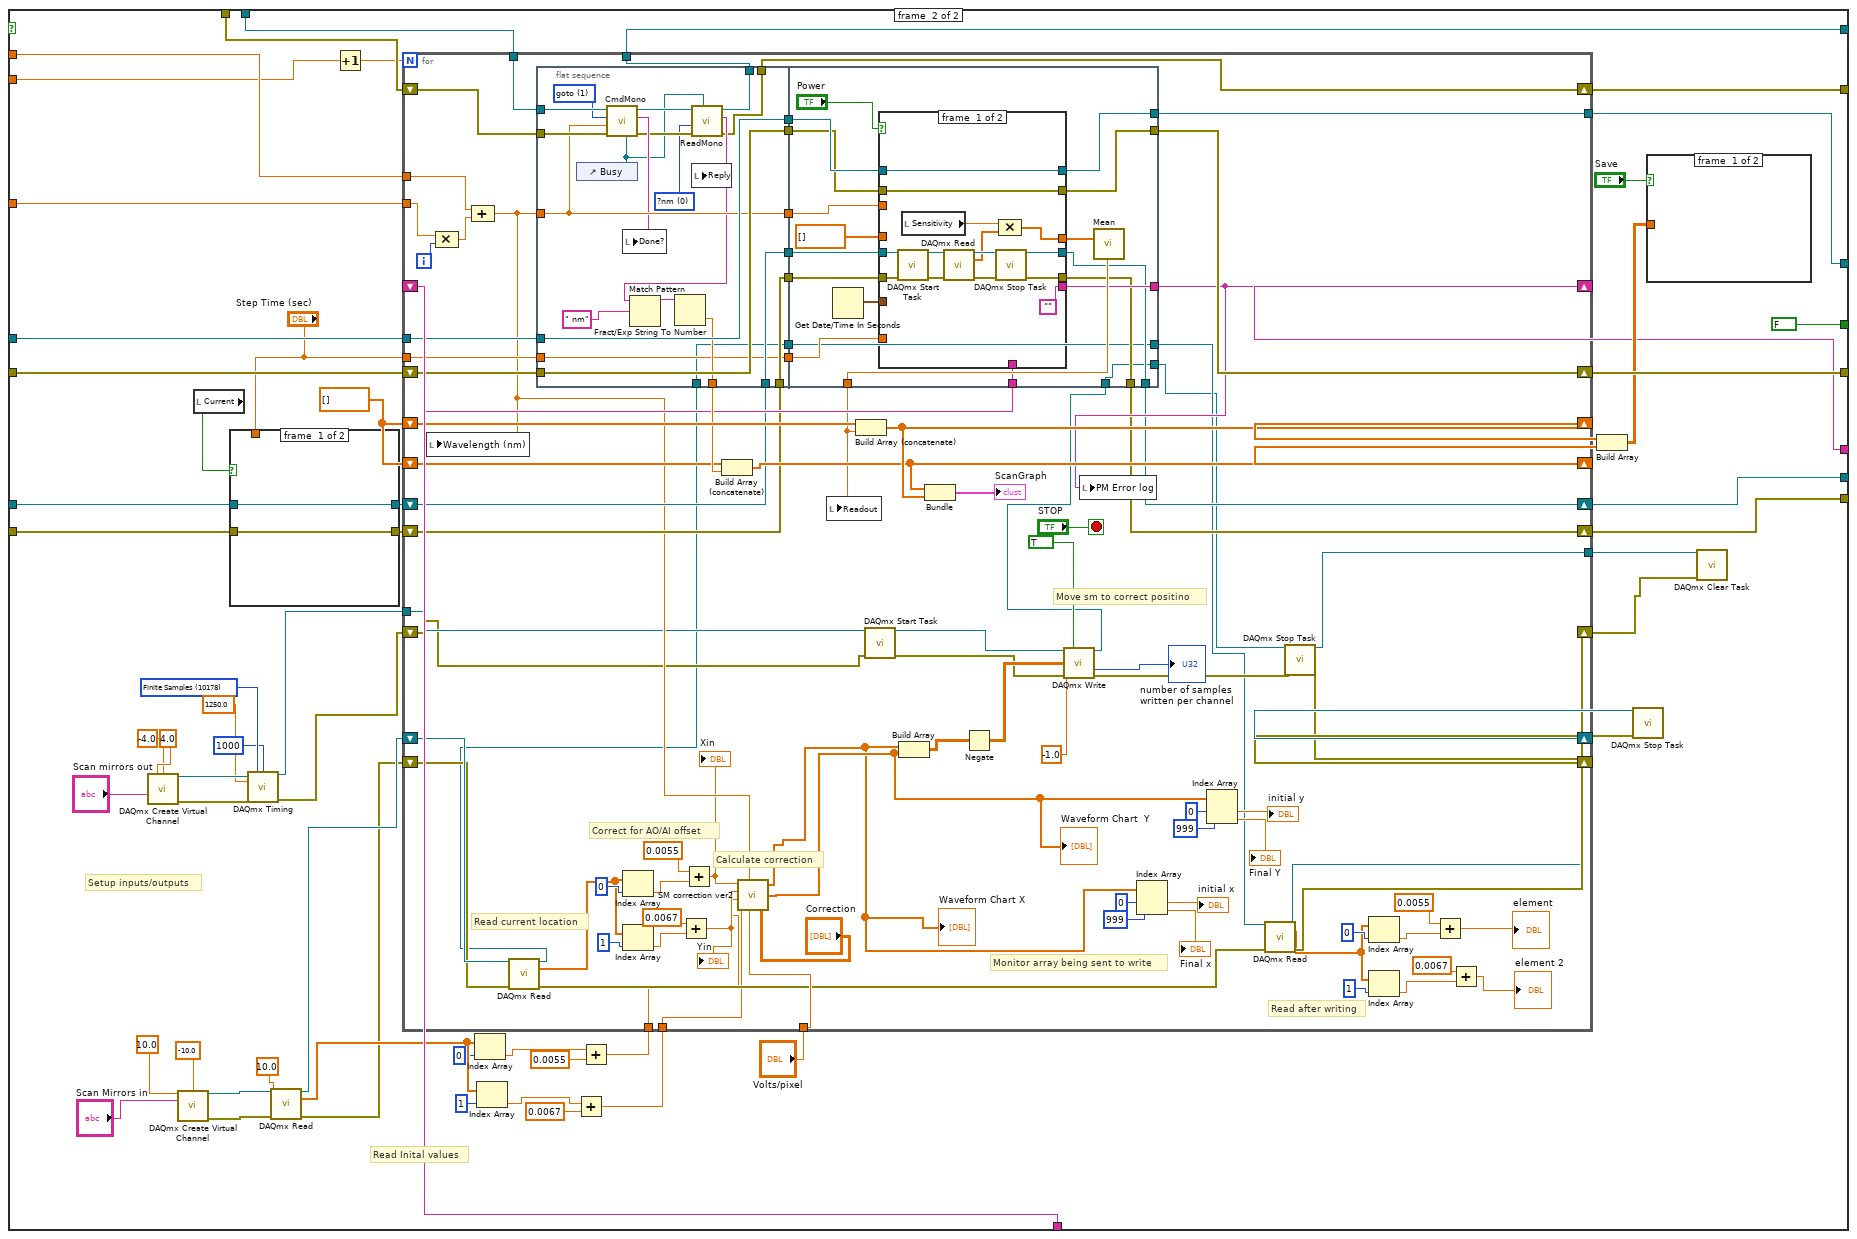
[diagram p15: hidden frame]
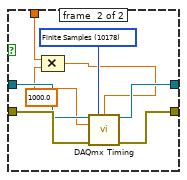
[diagram p16: hidden frame]
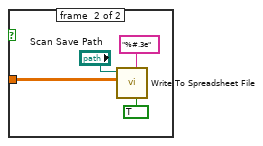
[diagram p17: hidden frame]
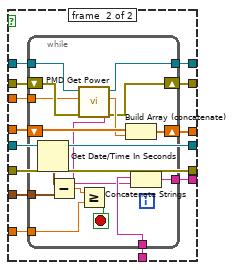
[diagram p18: hidden frame]
diagram:
  n1 = flat-sequence {
    tunnel: [w39] -> w20
    tunnel: [w38] -> w19
    tunnel: [w37] -> w18
    tunnel: [w36] -> w17
    tunnel: [w23] -> w12
    tunnel: [w24] -> w9
    tunnel: [w29] -> w8
    tunnel: [w30] -> w7
    tunnel: [w28] -> w6
    tunnel: [w27] -> w5
    tunnel: w20 -> [w64]
    tunnel: w19 -> [w65]
    tunnel: w18 -> [w63]
    tunnel: w17 -> [w62]
    tunnel: [w61] -> w16
    tunnel: [w60] -> w15
    tunnel: [w59] -> w14
    tunnel: [w58] -> w13
    tunnel: w12 -> [w55]
    tunnel: [w46] -> w11
    tunnel: [w45] -> w10
    tunnel: w9 -> [w56]
    tunnel: w8 -> [w54]
    tunnel: w7 -> [w53]
    tunnel: w6 -> [w52]
    tunnel: w5 -> [w51]
    tunnel: [w47] -> w4
    tunnel: [w48] -> w3
    tunnel: [w49] -> w2
    tunnel: [w50] -> w1
    tunnel: w16 -> [w526]
    tunnel: w15 -> [w525]
    tunnel: w14 -> [w524]
    tunnel: w13 -> [w523]
    tunnel: w11 -> [w521]
    tunnel: w10 -> [w522]
    tunnel: w4 -> [w520]
    tunnel: w3 -> [w519]
    tunnel: w2 -> [w518]
    tunnel: w1 -> [w517]
    frame #0 {
      w25 = -10.0 ("minimum value")
      w26 = 10.0 ("maximum value")
      n2 = call "PM100D_Initialize.vi"() -> ("error out"=w43:errorcluster, "Instrument"=→"IDN String":string, "VISA out"=w44:refnum<visa-resource-name>)  [unwired: 2 in, 1 out]
      n3 = call-poly <vilib>:"DAQmx Create Virtual Channel.vi"("maximum value"=w26, "minimum value"=w25, "physical channels"="Output A") -> ("task out"=w30:refnum<k21>, "error out"=w29:errorcluster)  [unwired: 11 in]
      n4 = call-poly <vilib>:"DAQmx Create Virtual Channel.vi"("maximum value"=10.0, "minimum value"=-10.0, "physical channels"="Input Channel") -> ("task out"=w24:refnum<k21>, "error out"=w23:errorcluster)  [unwired: 11 in]
      n5 = call "PM100D_SensorFlag.vi"("error in (no error)"=w43, "VISA in"=w44) -> ("error out"=w39:errorcluster, "VISA out"=w38:refnum<visa-resource-name>, "sn"=→"Sensor SN":string, "name"=→"Sensor Name":string)  [unwired: 2 in, 4 out]
      n6 = call-poly <vilib>:"DAQmx Create Virtual Channel.vi"("maximum value"=w26, "minimum value"=w25, "physical channels"="Output B") -> ("task out"=w27:refnum<k21>, "error out"=w28:errorcluster)  [unwired: 11 in]
      n7 = call "OpenMono.vi"("Mono Port"="Mono Port") -> ("VISA resource name out"=w37:refnum<visa-resource-name>, "error out"=w36:errorcluster)
      "Busy" <- FALSE ("Busy")
    }
    frame #1 {
      n8 = while {
        tunnel: w65 -> [w86]
        tunnel: w63 -> [w88]
        tunnel: [w83] -> w60
        tunnel: [w81] -> w58
        shift-right: [w80] -> w59
        shift-left: w64 -> [w85]
        shift-right: [w82] -> w61
        shift-left: w62 -> [w87]
        shift-right: [w78] -> _
        shift-left: "" -> [w79]
        shift-right: [w67] -> w45
        shift-left: w55 -> [w76]
        shift-right: [w66] -> w46
        shift-left: w56 -> [w77]
        shift-right: [w68] -> w50
        shift-left: w53 -> [w75]
        shift-right: [w69] -> w49
        shift-left: w54 -> [w74]
        shift-right: [w70] -> w48
        shift-left: w51 -> [w72]
        shift-right: [w71] -> w47
        shift-left: w52 -> [w73]
        stop <- "Exit" stop-if-true
        n9 = stacked-sequence {
          seq-local: [w107 _ _] -> [_ w203 _]
          seq-local: [w112 _ _] -> [_ _ w256]
          seq-local: [w111 _ _] -> [_ _ w255]
          seq-local: [_ w210 _] -> [_ _ w254]
          seq-local: [_ w211 _] -> [_ _ w253]
          seq-local: [_ w204 _] -> [_ _ w247]
          seq-local: [_ w198 _] -> [_ _ w243]
          seq-local: [_ w199 _] -> [_ _ w242]
          tunnel: w88 -> [w118 _ _]
          tunnel: w87 -> [w117 _ _]
          tunnel: w86 -> [_ w213 _]
          tunnel: w85 -> [_ w212 _]
          tunnel: [_ _ w252] -> w83
          tunnel: [_ _ w251] -> w82
          tunnel: [_ _ w250] -> w81
          tunnel: [_ _ w249] -> w80
          tunnel: w79 -> [_ w206 _]
          tunnel: [_ _ w246] -> w78
          tunnel: w77 -> [_ w197 _]
          tunnel: w76 -> [_ w196 _]
          tunnel: [_ _ w245] -> w66
          tunnel: [_ _ w244] -> w67
          tunnel: w75 -> [w102 _ _]
          tunnel: w74 -> [w103 _ _]
          tunnel: w73 -> [w105 _ _]
          tunnel: w72 -> [w104 _ _]
          tunnel: [w101 _ _] -> w71
          tunnel: [w100 _ _] -> w70
          tunnel: [w99 _ _] -> w69
          tunnel: [w98 _ _] -> w68
          frame #0 {
            # "Wavelength"
            n10 = while {
              shift-right: [w140] -> w89
              shift-left: _ -> [w139]
              tunnel: "Voltage B" -> [w140]
              tunnel: [w139] -> w94
              tunnel: "Voltage A" -> [w138]
              shift-right: [w138] -> w90
              shift-left: _ -> [w137]
              tunnel: [w137] -> w95
              stop <- TRUE stop-if-true
            }
            n11 = case shown="False" "Send Question" {
              tunnel: w118 -> [w188 w194]
              tunnel: w117 -> [w187 w193]
              tunnel: [w188 w192] -> w120
              tunnel: [w187 w191] -> w119
              frame #0 {
                (unwired) FALSE ("Read Error")
              }
              frame #1 {
                n12 = control-ref of="Busy"() -> (w189:refnum<vi>)
                n13 = call "ReadMono.vi"("Busy"=w189, "error in (no error)"=w193, "Cmd"="Ask?", "Mono Port"=w194) -> ("error out"=w191:errorcluster, "Response"=→"Reply":string, "Mono Port Out"=w192:refnum<visa-resource-name>)  [unwired: 2 in, 1 out]
              }
            }
            n14 = Not Equal?(x=w90, y=w95) -> (x != y?=w93:bool)
            n15 = Not Equal?(x=w89, y=w94) -> (x != y?=w92:bool)
            n16 = Or(x=w93, y=w92) -> (x .or. y?=w91:bool)
            n17 = case shown="False" w91 {
              tunnel: w105 -> [w123 w136]
              tunnel: w104 -> [w124 w135]
              tunnel: w103 -> [w125 w134]
              tunnel: w102 -> [w126 w133]
              tunnel: [w123 w132] -> w101
              tunnel: [w124 w131] -> w100
              tunnel: [w125 w130] -> w99
              tunnel: [w126 w129] -> w98
              tunnel: w90 -> [_ w127]
              tunnel: w89 -> [_ w128]
              frame #0 {
              }
              frame #1 {
                n18 = call-poly <vilib>:"DAQmx Write.vi"("task/channels in"=w135, "data"=w128, "error in"=w136) -> ("task out"=w131:refnum<k21>, "error out"=w132:errorcluster)  [unwired: 10 in, 1 out]
                n19 = call-poly <vilib>:"DAQmx Write.vi"("task/channels in"=w133, "data"=w127, "error in"=w134) -> ("task out"=w129:refnum<k21>, "error out"=w130:errorcluster)  [unwired: 10 in, 1 out]
              }
            }
            n20 = case shown="False" "Send Command" {
              tunnel: w120 -> [w173 w186]
              tunnel: w119 -> [w172 w185]
              tunnel: [w173 w178] -> w115
              tunnel: [w172 w177] -> w114
              tunnel: "Wavelength (nm)" -> [w171 w181]
              tunnel: [w171 w181] -> w113
              frame #0 {
              }
              frame #1 {
                w176 = u16 0 items=["?nm", "?nm/min", "?grating", "?turret", "?gratings"] ("Cmd")
                n21 = control-ref of="Busy"() -> (w174:refnum<vi>)
                n22 = call "CmdMono.vi"("Busy"=w174, "Scan Speed (nm/min)"="Scan Speed (nm/min)", "error in (no error)"=w185, "Wavelength (nm)"=w181, "Cmd"="Command", "Mono Port"=w186) -> ("error out"=w179:errorcluster, "Response"=→"Done?":string, "Mono Port Out"=w180:refnum<visa-resource-name>)  [unwired: 2 in, 1 out]
                n23 = call "ReadMono.vi"("Busy"=w174, "error in (no error)"=w179, "Cmd"=w176, "Mono Port"=w180) -> ("error out"=w177:errorcluster, "Response"=w175:string, "Mono Port Out"=w178:refnum<visa-resource-name>)  [unwired: 2 in, 1 out]
                n24 = local write "Reply"(w175) -> ()
              }
            }
            n25 = case shown="False" "Step" {
              tunnel: w115 -> [w151 w170]
              tunnel: w114 -> [w150 w169]
              tunnel: w113 -> [w149 w163]
              tunnel: [w151 w156] -> w112
              tunnel: [w150 w157] -> w111
              tunnel: "Increment (nm)" -> [_ w162]
              tunnel: [w149 w152] -> w107
              frame #0 {
              }
              frame #1 {
                w154 = u16 0 items=["?nm", "?nm/min", "?grating", "?turret", "?gratings"] ("Cmd")
                w161 = u16 1 items=["nm", "goto", "nm/min", "VIS grating", "IR grating"] ("Cmd")
                n26 = Select(t=1, s="Up", f=-1) -> (s? t:f=w168:i32)
                n27 = control-ref of="Busy"() -> (w153:refnum<vi>)
                n28 = Compound Arithmetic op=MULTIPLY(w168, w162) -> (w164:dbl)
                n29 = Compound Arithmetic op=ADD(w164, w163) -> (w152:dbl)
                n30 = call "CmdMono.vi"("Busy"=w153, "error in (no error)"=w169, "Wavelength (nm)"=w152, "Cmd"=w161, "Mono Port"=w170) -> ("error out"=w158:errorcluster, "Response"=w160:string, "Mono Port Out"=w159:refnum<visa-resource-name>)  [unwired: 3 in, 1 out]
                n31 = call "ReadMono.vi"("Busy"=w153, "error in (no error)"=w158, "Cmd"=w154, "Mono Port"=w159) -> ("error out"=w157:errorcluster, "Response"=w155:string, "Mono Port Out"=w156:refnum<visa-resource-name>)  [unwired: 2 in, 1 out]
                n32 = local write "Done?"(w160) -> ()
                n33 = local write "Reply"(w155) -> ()
              }
            }
            n34 = event shown="[0] Timeout" {
              selector: _ -> [_ _]
              dyn-events: _ -> [_ _]
              timeout: 0 -> [_ _]
              event #0 {
                n35 = event-data() -> ()  [unwired: 1 in, 2 out]
              }
              event #1 {
                n36 = event-data() -> ()  [unwired: 1 in, 1 out]
                n37 = local write "Done?"("   ..." ("Done?")) -> ()
              }
            }
            n38 = event shown="[0] Timeout" {
              selector: _ -> [_ _ _]
              dyn-events: _ -> [_ _ _]
              timeout: 0 -> [_ _ _]
              event #0 {
                n39 = event-data() -> ()  [unwired: 1 in, 2 out]
              }
              event #1 {
                n40 = event-data() -> ()  [unwired: 1 in, 7 out]
                n41 = local read "Power"() -> (w142:bool)
                n42 = case shown="False" w142 {
                  selector: w142 -> [w144 _]
                  frame #0 {
                    w143 = "Power (W)" ("Y Scale.Name Label.Text")
                    n43 = local write "Current"(w144) -> ()
                    n44 = property on="ScanGraph" class="XYGraph (strict)"("YScale.NameLbl.Text"=w143) -> ()  [unwired: 2 in, 2 out]
                    n45 = property on="Waveform Chart" class="WFChart (strict)"("YScale.NameLbl.Text"=w143) -> ()  [unwired: 2 in, 2 out]
                  }
                  frame #1 {
                  }
                }
                n46 = event-data("Discard?"=w142) -> ()  [unwired: 1 in, 1 out]
              }
              event #2 {
                n47 = event-data() -> ()  [unwired: 1 in, 7 out]
                n48 = local read "Current"() -> (w145:bool)
                n49 = case shown="False" w145 {
                  selector: w145 -> [w146 _]
                  frame #0 {
                    w147 = "Current (A)" ("Y Scale.Name Label.Text")
                    n50 = local write "Power"(w146) -> ()
                    n51 = property on="ScanGraph" class="XYGraph (strict)"("YScale.NameLbl.Text"=w147) -> ()  [unwired: 2 in, 2 out]
                    n52 = property on="Waveform Chart" class="WFChart (strict)"("YScale.NameLbl.Text"=w147) -> ()  [unwired: 2 in, 2 out]
                  }
                  frame #1 {
                  }
                }
                n53 = event-data("Discard?"=w145) -> ()  [unwired: 1 in, 1 out]
              }
            }
          }
          frame #1 {
            # "Wavelength"
            n54 = control-ref of="Zero?"() -> (w208:refnum<vi>)
            n55 = call "PMD Settings.vi"("Visa In"=w213, "Zero?"=w208, "PMD Settings In"="PMD Settings", "Error In"=w212, "Range"="Range") -> ("AUTO?"=→"AUTO?":bool, "Rng"=→"Rng":string, "Visa Out"=w216:refnum<visa-resource-name>, "ZeroValue"=→"Zero Value":dbl, "PM Error log"=w207:string, "error out"=w215:errorcluster)
            n56 = local write "Wavelength (nm)"(w203) -> ()
            n57 = call "PMD Get Power.vi"("VISA In"=w216, "Wavelength (nm)"=w203, "error in"=w215) -> ("PMD Error"=w205:string, "VISA out"=w210:refnum<visa-resource-name>, "Readout value"=w202:dbl, "error out"=w211:errorcluster)  [unwired: 1 in, 2 out]
            n58 = case shown="False" "Current" {
              tunnel: w202 -> [w223 _]
              tunnel: w197 -> [w222 w226]
              tunnel: w196 -> [w221 w227]
              tunnel: [w223 w239] -> w200
              tunnel: [w221 w235] -> w198
              tunnel: [w222 w236] -> w199
              frame #0 {
              }
              frame #1 {
                w229 = 10178 items=["Finite Samples"=10178, "Continuous Samples"=10123, "Hardware Timed Single Point"=12522] ("sample mode")
                n59 = call-poly <vilib>:"DAQmx Timing.vi"("task/channels in"=w226, "sample mode"=w229, "samples per channel"=50, "rate"=1000.0, "error in"=w227) -> ("task out"=w225:refnum<k21>, "error out"=w224:errorcluster)  [unwired: 9 in]
                n60 = call <vilib>:"DAQmx Start Task.vi"("task/channels in"=w225, "error in"=w224) -> ("task out"=w237:refnum<k21>, "error out"=w238:errorcluster)  [unwired: 12 in]
                n61 = call-poly <vilib>:"DAQmx Read.vi"("task/channels in"=w237, "error in"=w238) -> ("task out"=w233:refnum<k21>, "data"=w232:dbl[], "error out"=w234:errorcluster)  [unwired: 11 in]
                n62 = call <vilib>:"Mean.vi"("X"=w232) -> ("mean"=w231:dbl)  [unwired: 1 out]
                n63 = Compound Arithmetic op=MULTIPLY("Sensitivity", w231) -> (w239:dbl)
                n64 = call <vilib>:"DAQmx Stop Task.vi"("task/channels in"=w233, "error in"=w234) -> ("task out"=w236:refnum<k21>, "error out"=w235:errorcluster)  [unwired: 12 in]
              }
            }
            "Readout" <- w200
            n65 = Concatenate Strings(w206, w207, w205) -> (w204:string)
            n66 = case shown="False" "On" {
              tunnel: w200 -> [_ w241]
              frame #0 {
              }
              frame #1 {
                "Waveform Chart" <- w241
              }
            }
          }
          frame #2 {
            # "Wavelength"
            n67 = Subtract(x="End", y="Start") -> (x-y=w261:dbl)
            n68 = Divide(x=w261, y="Step Size (nm)") -> (x/y=w260:dbl)
            n69 = Round To Nearest(number=w260) -> (nearest integer value=w259:dbl)
            n70 = case shown="True" "Scan" {
              tunnel: w259 -> [_ w326]
              tunnel: w255 -> [w269 w328]
              tunnel: w256 -> [w268 w329]
              tunnel: "Start" -> [_ w331]
              tunnel: "Step Size (nm)" -> [_ w330]
              tunnel: w254 -> [w271 w324]
              tunnel: w253 -> [w270 w323]
              tunnel: [w271 w312] -> w250
              tunnel: [w270 w322] -> w249
              tunnel: [w269 w321] -> w251
              tunnel: [w268 w320] -> w252
              tunnel: [FALSE ("Scan") FALSE ("Scan")] -> w248
              tunnel: w247 -> [w266 w314]
              tunnel: [w266 w313] -> w246
              tunnel: [w265 w311] -> w245
              tunnel: [w264 w310] -> w244
              tunnel: w243 -> [w264 w308]
              tunnel: w242 -> [w265 w307]
              frame #0 {
              }
              frame #1 {
                w283 = 10178 items=["Finite Samples"=10178, "Continuous Samples"=10123, "Hardware Timed Single Point"=12522] ("sample mode")
                w327 = dbl[] []
                # "Read Inital values"
                # "Setup inputs/outputs"
                n71 = call-poly <vilib>:"DAQmx Create Virtual Channel.vi"("maximum value"=4.0, "minimum value"=-4.0, "physical channels"="Scan mirrors out") -> ("task out"=w291:refnum<k21>, "error out"=w290:errorcluster)  [unwired: 11 in]
                n72 = call-poly <vilib>:"DAQmx Create Virtual Channel.vi"("maximum value"=10.0, "minimum value"=-10.0, "physical channels"="Scan Mirrors in") -> ("task out"=w298:refnum<k21>, "error out"=w302:errorcluster)  [unwired: 11 in]
                n73 = local read "Current"() -> (w309:bool)
                n74 = case shown="False" w309 {
                  tunnel: w308 -> [w332 w340]
                  tunnel: w307 -> [w333 w339]
                  tunnel: [w333 w338] -> w306
                  tunnel: [w332 w337] -> w305
                  tunnel: "Step Time (sec)" -> [_ w336]
                  frame #0 {
                  }
                  frame #1 {
                    w341 = 10178 items=["Finite Samples"=10178, "Continuous Samples"=10123, "Hardware Timed Single Point"=12522] ("sample mode")
                    w335 = 1000.0 ("rate")
                    n75 = Compound Arithmetic op=MULTIPLY(w336, w335) -> (w334:dbl)
                    n76 = call-poly <vilib>:"DAQmx Timing.vi"("task/channels in"=w339, "sample mode"=w341, "samples per channel"=w334, "rate"=w335, "error in"=w340) -> ("task out"=w338:refnum<k21>, "error out"=w337:errorcluster)  [unwired: 9 in]
                  }
                }
                n77 = call-poly <vilib>:"DAQmx Timing.vi"("task/channels in"=w291, "sample mode"=w283, "samples per channel"=1000, "rate"=1250.0, "error in"=w290) -> ("task out"=w280:refnum<k21>, "error out"=w281:errorcluster)  [unwired: 9 in]
                n78 = call-poly <vilib>:"DAQmx Read.vi"("task/channels in"=w298, "timeout"=10.0, "error in"=w302) -> ("task out"=w289:refnum<k21>, "data"=w297:dbl[], "error out"=w288:errorcluster)  [unwired: 10 in]
                n79 = Increment(x=w326) -> (x+1=w325:dbl)
                n80 = Index Array(array=w297, index=0) -> (element=w274:dbl)
                n81 = Index Array(array=w297, index=1) -> (element=w276:dbl)
                n82 = Add(x=w276, y=0.0067) -> (x+y=w275:dbl)
                n83 = Add(x=w274, y=0.0055) -> (x+y=w272:dbl)
                n84 = for {
                  N: w325 -> [_]
                  tunnel: w329 -> [w431]
                  tunnel: w331 -> [w427]
                  tunnel: w330 -> [w429]
                  shift-right: [w415] -> w319
                  shift-left: w327 -> [w433]
                  shift-right: [w426] -> w321
                  shift-left: w328 -> [w432]
                  shift-right: [w412] -> w318
                  shift-left: w327 -> [w413]
                  tunnel: w324 -> [w424]
                  shift-right: [w419] -> w322
                  shift-left: w323 -> [w423]
                  tunnel: [w418] -> w312
                  tunnel: [w417] -> w320
                  shift-right: [w410] -> w313
                  shift-left: w314 -> [w411]
                  shift-right: [w407] -> w310
                  shift-left: w305 -> [w402]
                  shift-right: [w406] -> w311
                  shift-left: w306 -> [w403]
                  tunnel: "Step Time (sec)" -> [w404]
                  tunnel: w272 -> [w356]
                  tunnel: w275 -> [w357]
                  shift-right: [w386] -> w278
                  shift-left: w281 -> [w384]
                  shift-right: [w376] -> w287
                  shift-left: w289 -> [w397]
                  shift-right: [w377] -> w286
                  shift-left: w288 -> [w396]
                  tunnel: "Volts/pixel" -> [w393]
                  tunnel: w280 -> [w385]
                  tunnel: [w346] -> w279
                  i -> [w430]
                  stop <- "STOP" stop-if-true
                  # "Move sm to correct positino"
                  # "Monitor array being sent to write"
                  # "Read after writing"
                  # "Calculate correction"
                  # "Correct for AO/AI offset"
                  # "Read current location"
                  n85 = Compound Arithmetic op=MULTIPLY(w429, w430) -> (w428:dbl)
                  n86 = Compound Arithmetic op=ADD(w427, w428) -> (w395:dbl)
                  n87 = local write "Wavelength (nm)"(w395) -> ()
                  n88 = call-poly <vilib>:"DAQmx Read.vi"("task/channels in"=w397, "error in"=w396) -> ("task out"=w351:refnum<k21>, "data"=w398:dbl[], "error out"=w378:errorcluster)  [unwired: 11 in]
                  n89 = flat-sequence {
                    tunnel: w432 -> [w454]
                    tunnel: w431 -> [w453]
                    tunnel: w395 -> [w449]
                    tunnel: [w438] -> w426
                    tunnel: w424 -> [w451]
                    tunnel: w423 -> [w450]
                    tunnel: [w451] -> w422
                    tunnel: [w450] -> w421
                    tunnel: [w449] -> w420
                    tunnel: [w443] -> w417
                    tunnel: [w439] -> w414
                    tunnel: w402 -> [w436]
                    tunnel: [w437] -> w409
                    tunnel: w403 -> [w437]
                    tunnel: [w436] -> w408
                    tunnel: [w435] -> w405
                    tunnel: w404 -> [w435]
                    tunnel: w351 -> [w434]
                    tunnel: [w434] -> w350
                    tunnel: [w470] -> w401
                    tunnel: w422 -> [w469]
                    tunnel: w421 -> [w468]
                    tunnel: w420 -> [w467]
                    tunnel: [w463] -> w419
                    tunnel: [w466] -> w418
                    tunnel: w411 -> [w465]
                    tunnel: [w464] -> w410
                    tunnel: w409 -> [w461]
                    tunnel: w408 -> [w460]
                    tunnel: [w458] -> w406
                    tunnel: [w459] -> w407
                    tunnel: w405 -> [w462]
                    tunnel: w348 -> [w456]
                    tunnel: [w456] -> w347
                    tunnel: [w455] -> w349
                    tunnel: w350 -> [w455]
                    frame #0 {
                      w445 = u16 0 items=["?nm", "?nm/min", "?grating", "?turret", "?gratings"] ("Cmd")
                      w452 = u16 1 items=["nm", "goto", "nm/min", "VIS grating", "IR grating"] ("Cmd")
                      n90 = control-ref of="Busy"() -> (w444:refnum<vi>)
                      n91 = call "CmdMono.vi"("Busy"=w444, "error in (no error)"=w454, "Wavelength (nm)"=w449, "Cmd"=w452, "Mono Port"=w453) -> ("error out"=w446:errorcluster, "Response"=w448:string, "Mono Port Out"=w447:refnum<visa-resource-name>)  [unwired: 3 in, 1 out]
                      n92 = local write "Done?"(w448) -> ()
                      n93 = call "ReadMono.vi"("Busy"=w444, "error in (no error)"=w446, "Cmd"=w445, "Mono Port"=w447) -> ("error out"=w438:errorcluster, "Response"=w441:string, "Mono Port Out"=w443:refnum<visa-resource-name>)  [unwired: 2 in, 1 out]
                      n94 = Match Pattern(string=w441, regular expression=" nm") -> (before substring=w440:string)  [unwired: 1 in, 3 out]
                      n95 = Fract/Exp String To Number(string=w440) -> (number=w439:dbl)  [unwired: 3 in, 1 out]
                      n96 = local write "Reply"(w441) -> ()
                    }
                    frame #1 {
                      n97 = Get Date/Time In Seconds() -> (seconds since 1Jan1904=w472:timestamp)
                      n98 = case shown="True" "Power" {
                        tunnel: dbl[] [] -> [_ w500]
                        tunnel: w472 -> [_ w499]
                        tunnel: [w474 w498] -> w471
                        tunnel: w469 -> [w486 w497]
                        tunnel: w468 -> [w485 w496]
                        tunnel: w467 -> [_ w495]
                        tunnel: [w486 w494] -> w466
                        tunnel: w465 -> [_ w493]
                        tunnel: ["" w492] -> w464
                        tunnel: [w485 w491] -> w463
                        tunnel: w462 -> [_ w490]
                        tunnel: w461 -> [w484 w488]
                        tunnel: w460 -> [w483 w489]
                        tunnel: [w478 w489] -> w459
                        tunnel: [w477 w488] -> w458
                        frame #0 {
                          n99 = call <vilib>:"DAQmx Start Task.vi"("task/channels in"=w484, "error in"=w483) -> ("task out"=w482:refnum<k21>, "error out"=w481:errorcluster)  [unwired: 12 in]
                          n100 = local read "Sensitivity"() -> (w475:dbl)
                          n101 = call-poly <vilib>:"DAQmx Read.vi"("task/channels in"=w482, "error in"=w481) -> ("task out"=w480:refnum<k21>, "data"=w476:dbl[], "error out"=w479:errorcluster)  [unwired: 11 in]
                          n102 = call <vilib>:"DAQmx Stop Task.vi"("task/channels in"=w480, "error in"=w479) -> ("task out"=w477:refnum<k21>, "error out"=w478:errorcluster)  [unwired: 12 in]
                          n103 = Compound Arithmetic op=MULTIPLY(w475, w476) -> (w474:dbl[])
                        }
                        frame #1 {
                          n104 = while {
                            shift-right: [w515] -> w498
                            shift-left: w500 -> [w516]
                            tunnel: w499 -> [w513]
                            tunnel: w497 -> [w508]
                            tunnel: w495 -> [w504]
                            tunnel: [w506] -> w494
                            tunnel: w493 -> [w510]
                            tunnel: [w509] -> w492
                            shift-right: [w502] -> w491
                            shift-left: w496 -> [w507]
                            tunnel: w490 -> [w501]
                            stop <- w511 stop-if-true
                            n105 = Get Date/Time In Seconds() -> (seconds since 1Jan1904=w514:timestamp)
                            n106 = Subtract(x=w514, y=w513) -> (x-y=w512:dbl)
                            n107 = call "PMD Get Power.vi"("VISA In"=w508, "Wavelength (nm)"=w504, "error in"=w507) -> ("PMD Error"=w503:string, "VISA out"=w506:refnum<visa-resource-name>, "Readout value"=w505:dbl, "error out"=w502:errorcluster)  [unwired: 1 in, 2 out]
                            n108 = Greater Or Equal?(x=w512, y=w501) -> (x >= y?=w511:bool)
                            n109 = Build Array (concatenate)(w516, w505) -> (w515:dbl[])
                            n110 = Concatenate Strings(w510, w503) -> (w509:string)
                          }
                        }
                      }
                      n111 = call <vilib>:"Mean.vi"("X"=w471) -> ("mean"=w470:dbl)  [unwired: 1 out]
                    }
                  }
                  n112 = Index Array(array=w398, index=0) -> (element=w369:dbl)
                  n113 = Index Array(array=w398, index=1) -> (element=w366:dbl)
                  n114 = Add(x=0.0067, y=w366) -> (x+y=w364:dbl)
                  "Yin" <- w364
                  n115 = Add(x=0.0055, y=w369) -> (x+y=w367:dbl)
                  "Xin" <- w367
                  n116 = Build Array (concatenate)(w413, w414) -> (w412:dbl[])
                  n117 = call "SM correction ver2.vi"("V in x"=w367, "nm in"=w395, "V in y"=w364, "V x initial"=w356, "Volts/pixel"=w393, "V y initial"=w357, "Array"="Correction") -> ("V out x"=w370:dbl[], "V out y"=w379:dbl[])
                  "Waveform Chart X" <- w370
                  "Waveform Chart  Y" <- w379
                  n118 = local write "Readout"(w401) -> ()
                  n119 = Build Array (concatenate)(w433, w401) -> (w415:dbl[])
                  n120 = call <vilib>:"DAQmx Start Task.vi"("task/channels in"=w385, "error in"=w384) -> ("task out"=w354:refnum<k21>, "error out"=w353:errorcluster)  [unwired: 12 in]
                  n121 = Build Array(w370, w379) -> (w372:dbl[][])
                  n122 = Bundle(w412, w415) -> (→"ScanGraph":cluster{dbl[], dbl[]})  [unwired: 1 in]
                  n123 = Negate(x=w372) -> (-x=w371:dbl[][])
                  n124 = call-poly <vilib>:"DAQmx Write.vi"("task/channels in"=w354, "auto start"=TRUE, "data"=w371, "timeout"=-1.0, "error in"=w353) -> ("task out"=w348:refnum<k21>, "number of samples written per channel"=→"number of samples written per channel":u32, "error out"=w355:errorcluster)  [unwired: 8 in]
                  n125 = local write "PM Error log"(w410) -> ()
                  n126 = Index Array(array=w370, index #1=0 ("index"), index #2=999 ("index")) -> (element #1=→"initial x":dbl, element #2=→"Final x":dbl)
                  n127 = Index Array(array=w379, index #1=0 ("index"), index #2=999 ("index")) -> (element #1=→"initial y":dbl, element #2=→"Final Y":dbl)
                  n128 = call-poly <vilib>:"DAQmx Read.vi"("task/channels in"=w349, "error in"=w378) -> ("task out"=w376:refnum<k21>, "data"=w373:dbl[], "error out"=w377:errorcluster)  [unwired: 11 in]
                  n129 = call <vilib>:"DAQmx Stop Task.vi"("task/channels in"=w347, "error in"=w355) -> ("task out"=w346:refnum<k21>, "error out"=w386:errorcluster)  [unwired: 12 in]
                  n130 = Index Array(array=w373, index=0) -> (element=w360:dbl)
                  n131 = Index Array(array=w373, index=1) -> (element=w361:dbl)
                  n132 = Add(x=0.0055, y=w360) -> (x+y=→"element":dbl)
                  n133 = Add(x=0.0067, y=w361) -> (x+y=→"element 2":dbl)
                }
                n134 = Build Array(w319, w318) -> (w317:dbl[][])
                n135 = call <vilib>:"DAQmx Stop Task.vi"("task/channels in"=w287, "error in"=w286) -> ()  [unwired: 12 in, 2 out]
                n136 = case shown="False" "Save" {
                  tunnel: w317 -> [_ w342]
                  frame #0 {
                  }
                  frame #1 {
                    n137 = call-poly <vilib>:"Write To Spreadsheet File.vi"("transpose? (no:F)"=TRUE, "format (%.3f)"="%#.3e", "2D data"=w342, "file path (dialog if empty)"="Scan Save Path") -> ()  [unwired: 4 in, 1 out]
                  }
                }
                n138 = call <vilib>:"DAQmx Clear Task.vi"("task in"=w279, "error in"=w278) -> ()  [unwired: 13 in, 1 out]
              }
            }
            n139 = local write "Scan"(w248) -> ()
          }
        }
        "PM Error log" <- w78
      }
    }
    frame #2 {
      n140 = call <vilib>:"DAQmx Clear Task.vi"("task in"=w521, "error in"=w522) -> ()  [unwired: 13 in, 1 out]
      n141 = call <vilib>:"DAQmx Clear Task.vi"("task in"=w517, "error in"=w518) -> ()  [unwired: 13 in, 1 out]
      n142 = call <vilib>:"DAQmx Clear Task.vi"("task in"=w519, "error in"=w520) -> ()  [unwired: 13 in, 1 out]
      n143 = VISA Close(VISA resource name=w525, error in (no error)=w526) -> (error out=w527:errorcluster)
      n144 = call "PM100D_Close.vi"("error in (no error)"=w524, "VISA resource name"=w523) -> ()  [unwired: 2 in]
      n145 = call <vilib>:"Simple Error Handler.vi"("error in (no error)"=w527) -> ()  [unwired: 1 in, 8 out]
    }
  }
